vi "Main.vi"() -> ()   [LabVIEW 2018]
uses:
  TypeDefs/Enum_MainQueueElements.ctl
  TypeDefs/Refs_Common.ctl
  TypeDefs/Graph_DataArrayElement.ctl
  <vilib>/event_ctls.llb/eventvkey.ctl
  TypeDefs/TD_Case_SimpleFGVModes.ctl
  TypeDefs/Enum_CmdPromptActions.ctl
  TypeDefs/TD_Case_RecControll_DisableControlls.ctl
  OXYGEN/TypeDefs/Cluster_RawCommData.ctl
  TypeDefs/TD_Case_MeasurementValues.ctl
  OXYGEN/TypeDefs/Enum_ELOGtimeFormats.ctl
  TypeDefs/TD_Case_ELOG-ManageGUI.ctl
  OXYGEN/VIs/Common Commands/SubVIs/GetID.vi
  OXYGEN/VIs/Common Commands/SubVIs/GetSoftwareVersion.vi
  OXYGEN/VIs/Error Handling/SubVIs/ErrorHandling_GetError.vi
  OXYGEN/VIs/Application Control/SubVIs/ApplicationSetup_Load.vi
  OXYGEN/VIs/Recording Control/SubVIs/RecordingControl_SetFileName.vi
  OXYGEN/VIs/Channel List Access/SubVIs/ChannelList_GetNames.vi
  OXYGEN/VIs/Recording Control/SubVIs/RecordingControl_Start.vi
  OXYGEN/VIs/Recording Control/SubVIs/RecordingControl_Pause.vi
  OXYGEN/VIs/Recording Control/SubVIs/RecordingControl_Stop.vi
  OXYGEN/VIs/Measurement Values/SubVIs/AggregationRate_Set.vi
  OXYGEN/VIs/Measurement Values/SubVIs/MeasurementItems_SetChannels.vi
  OXYGEN/VIs/External Data Logging/SubVIs/ELOG_Channels_Set.vi
  OXYGEN/VIs/External Data Logging/SubVIs/ELOG_AggregationPeriod_Set.vi
  OXYGEN/VIs/External Data Logging/SubVIs/ELOG_Calculations_Set.vi
  OXYGEN/VIs/External Data Logging/SubVIs/ELOG_TimestampFormat_Set.vi
  OXYGEN/VIs/External Data Logging/SubVIs/ELOG_Control_Start.vi
  OXYGEN/VIs/External Data Logging/SubVIs/ELOG_Control_Stop.vi
  OXYGEN/VIs/External Data Logging/SubVIs/ELOG_Control_Reset.vi
  OXYGEN.lvlib
panel:
  out "Bool_StatusLED":bool=TRUE
  in  "STR_HostAddress":string
  in  "Button_Disconnect":bool
  in  "Button_Connect":bool
  in  "LBox_ChList":i32(listbox)
  in  "Tab_Selections":T1(tab)
  in  "Indicator_RecordingStatus":u32(colorbox)
  in  "STR_SetupSetFileName":path
  in  "STR_SetupLoadFileName":path
  in  "Button_Identification":bool
  in  "Button_Version":bool
  in  "Button_Reset":bool
  in  "Button_Error":bool
  in  "Button_LoadSetup":bool
  in  "Button_SetFileName":bool
  in  "Button_QuerryChList":bool
  in  "Button_StartRec":bool
  in  "Button_PauseRec":bool
  in  "Button_StopRec":bool
  in  "Button_UsrCmdSet":bool
  in  "STR_UserCommand":string
  in  "Button_AggregationRate":bool
  in  "STR_IN_AggregationRate":dbl=0.001 min=0.001 max=5.0 format="%.3p"
  in  "STR_ChName1":string
  out "Num_ChValue1":dbl format="%04.3g"
  in  "STR_ChName2":string
  out "Num_ChValue2":dbl format="%1.3g"
  in  "STR_ChName3":string
  out "Num_ChValue3":dbl format="%1.3g"
  in  "STR_ChName4":string
  out "Num_ChValue4":dbl format="%.3g"
  in  "STR_ChName5":string
  out "Num_ChValue5":dbl format="%.3g"
  in  "STR_ChName6":string
  out "Num_ChValue6":dbl format="%.3g"
  out "Recorder":T2(graph)
  in  "Button_StartTransfer":bool
  in  "Button_StopTransfer":bool
  in  "STR_LoggingChName3":string
  in  "STR_LoggingChName2":string
  in  "STR_LoggingChName4":string
  in  "STR_LoggingChName5":string
  in  "STR_LoggingChName6":string
  in  "Enum_SelectCalc":u16(ring) items=["AVG", "MIN", "MAX", "RMS"]
  in  "Enum_SelectTimestampFormat":u16(ring) items=["OFF", "REL", "ABS", "ELOG"]
  in  "Num_SetDurationTime":dbl=0.001 min=0.0001 max=30.0 format="%1.3p"
  in  "STR_LoggingChName1":string
  out "Listbox_ChValue":i32(listbox)
  out "RecoderLogging":T2(graph)
  in  "Button_StartBuffer":bool
  in  "Button_FetchData":bool
  in  "Button_StopBuffer":bool
  out "STR_CmdPrompt":string
  # "IP Address/Hostname and Port Number \n                Example:  xxx.xxx.xxx.xxx:Port"
  # "Common Commands"
  # "Setup Managment"
  # "Recording Control"
  # "User Command"
  # "s"
  # "Channel 1"
  # "Channel 3"
  # "Channel 2"
  # "Channel 5"
  # "Channel 4"
  # "Channel 6"
  # "Channel 1"
  # "Channel 2"
  # "Channel 3"
  # "Channel 4"
  # "Channel 5"
  # "Channel 6"
  # "Timestamp"
  # "Calculations"
  # "Period"
  # "s"
  # "Channel 1"
  # "Channel 2"
  # "Channel 3"
  # "Channel 4"
  # "Channel 5"
  # "Channel 6"
  # "Channel 1"
  # "Channel 2"
  # "Channel 3"
  # "Channel 4"
  # "Channel 5"
  # "Channel 6"
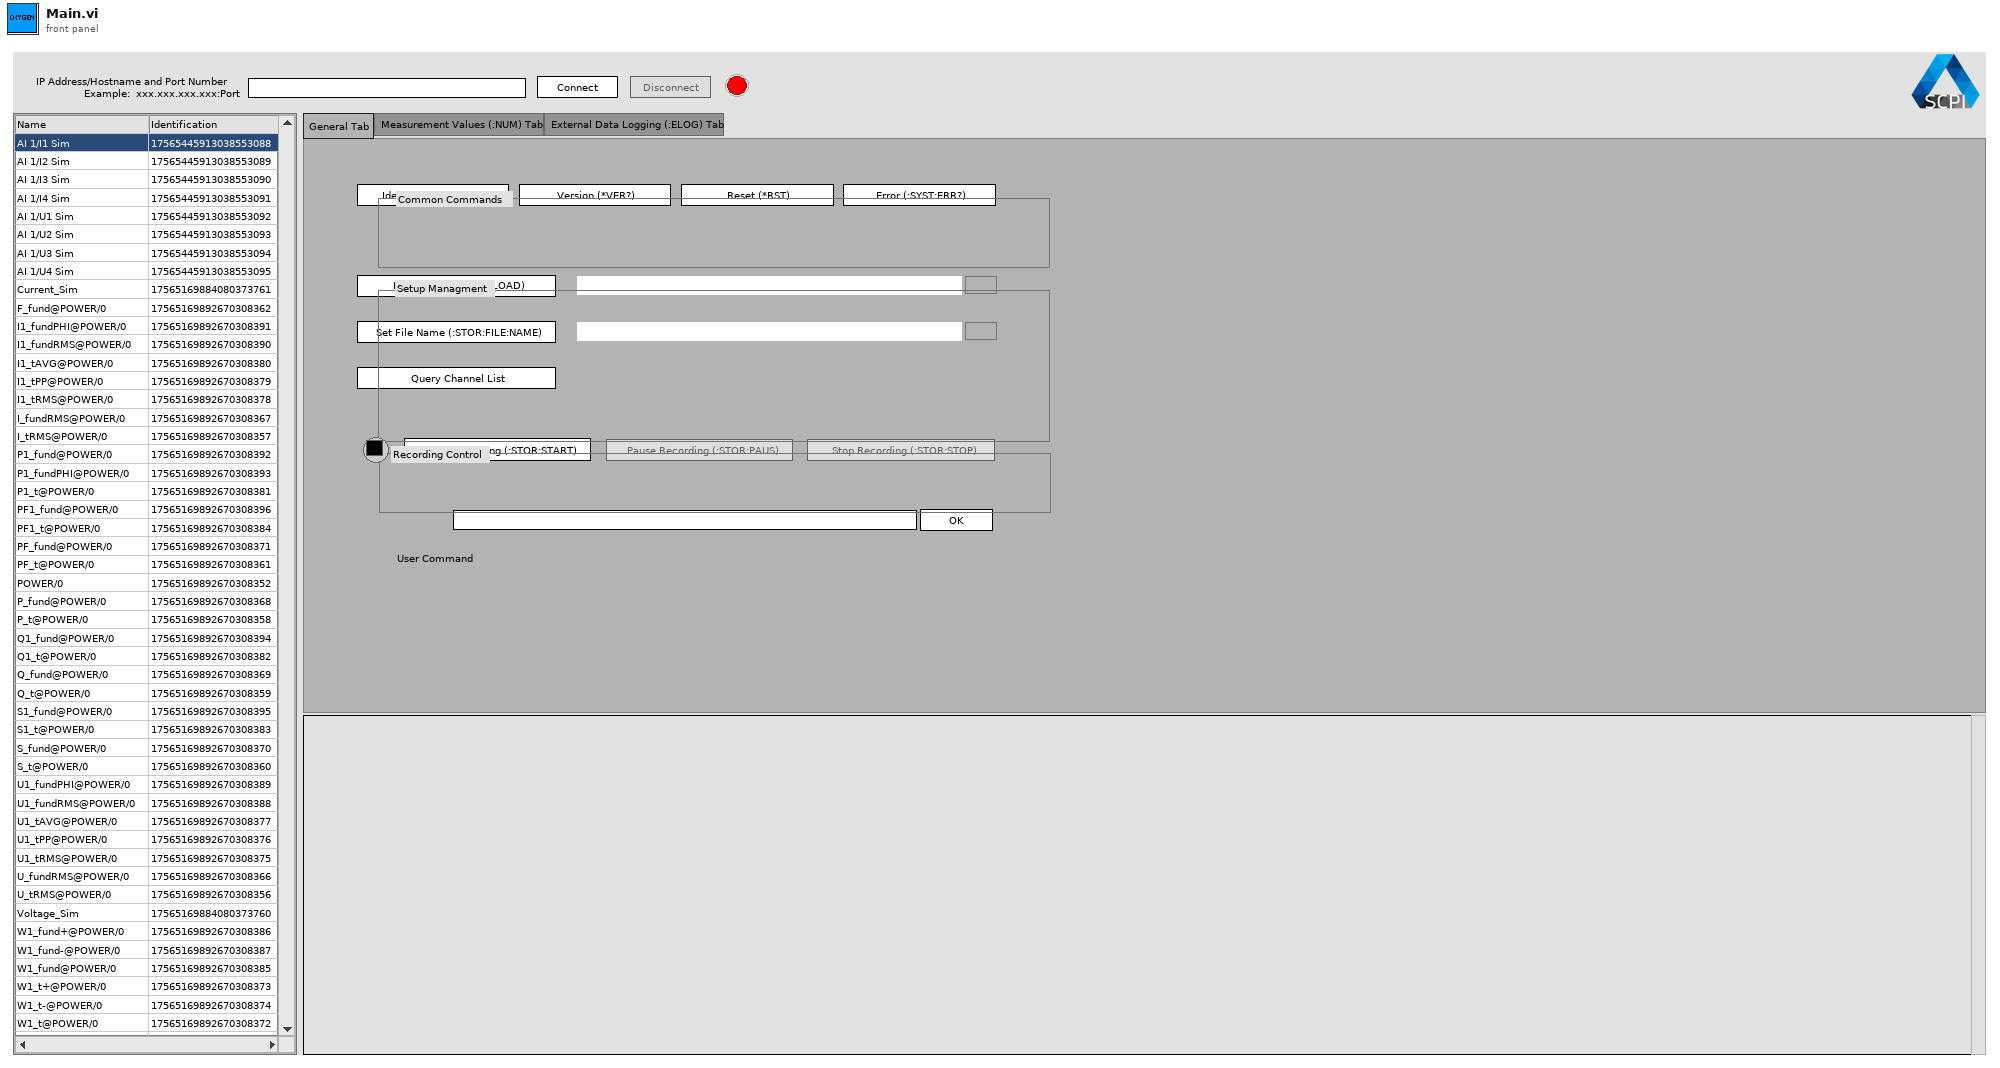
[diagram p1: front panel]
types:
  T1 = enum32{"General Tab", "Measurement Values (:NUM) Tab", "External Data Logging (:ELOG) Tab"}
  T2 = cluster{"Timestamp":timestamp[], "Value":dbl[]}[]
  T3 = typedef "Graph_DataArrayElement.ctl" = cluster{"Timestamp":timestamp[], "Value":dbl[]}
  T4 = typedef "Refs_Common.ctl" = cluster{"LBox_ChList":refnum<vi>, "STR_LoggingChName1":refnum<vi>, "Listbox_ChValue":refnum<vi>, "STR_LoggingChName2":refnum<vi>, "STR_LoggingChName3":refnum<vi>, "STR_LoggingChName4":refnum<vi>, "STR_LoggingChName5":refnum<vi>, "STR_LoggingChName6":refnum<vi>, "OXY_SCPI Ref":refnum<visa-resource-name>, "STR_ChName1":refnum<vi>, "STR_ChName2":refnum<vi>, "STR_ChName3":refnum<vi>, "STR_ChName4":refnum<vi>, "STR_ChName5":refnum<vi>, "STR_ChName6":refnum<vi>, "Enum_SelectTimestampFormat":refnum<vi>, "GRAPH-XY_ELOG":refnum<vi>, "GRAPH-XY_Measurement":refnum<vi>, "Button_StartBuffer":refnum<vi>, "Button_StopBuffer":refnum<vi>, "Button_FetchData":refnum<vi>, "STR_LoggingChName1":refnum<vi>, "STR_LoggingChName2":refnum<vi>, "STR_LoggingChName3":refnum<vi>, "STR_LoggingChName4":refnum<vi>, "STR_LoggingChName5":refnum<vi>, "STR_LoggingChName6":refnum<vi>, "Enum_SelectCalc":refnum<vi>, "Num_SetDurationTime":refnum<vi>, "Button_StopTransfer":refnum<vi>, "Button_StartTransfer":refnum<vi>, "STR_IN_AggregationRate":refnum<vi>, "Button_Disconnect":refnum<vi>, "Button_Connect":refnum<vi>, "Button_StartRec":refnum<vi>, "Button_PauseRec":refnum<vi>, "Button_StopRec":refnum<vi>, "Bool_StatusLED":refnum<vi>, "Indicator_RecordingStatus":refnum<vi>}
  T5 = typedef "Enum_MainQueueElements.ctl" = enum16{"Timeout", "Init", "Button_Identification_Pressed", "Button_Version_Pressed", "Button_Reset_Pressed", "Button_Error_Pressed", "Button_LoadSetup_Pressed", "Button_SetFileName_Pressed", "Button_QuerryChList_Pressed", "Button_StartRec_Pressed", "Button_PauseRec_Pressed", "Button_StopRec_Pressed", "Button_UsrCmdSet_Pressed", "Button_AggregationRate_Pressed", "Button_StartTransfer_Pressed", "Button_StopTransfer_Pressed", "Button_StartBuffer_Pressed", "Button_FetchData_Pressed", "Button_StopBuffer_Pressed", "Button_Connect_Pressed", "Button_Disconnect_Pressed", "NewDragAndDrop", "CloseApp"}
  T6 = typedef "Enum_CmdPromptActions.ctl" = enum16{"Init", "Add", "EditSettings", "Close"}
  T7 = typedef "TD_Case_RecControll_DisableControlls.ctl" = enum16{"Start", "Pause", "Stop"}
  T8 = typedef "OXYGEN.lvlib/Cluster_RawCommData.ctl" = cluster{"send_data":string, "received_data":string}
  T9 = typedef "TD_Case_MeasurementValues.ctl" = enum16{"Init", "Start", "Stop", "ChangeChannel", "Refresh"}
  T10 = typedef "OXYGEN.lvlib/Enum_ELOGtimeFormats.ctl" = enum16{"OFF", "REL", "ELOG", "ABS"}
  T11 = typedef "TD_Case_ELOG-ManageGUI.ctl" = enum16{"Reset", "AddDataToGUI"}
  T12 = enum8{"Enabled", "Disabled", "Disabled and Grayed Out"}
  T13 = typedef "TD_Case_SimpleFGVModes.ctl" = enum16{"Set", "Get"}
  T14 = typedef "OXYGEN.lvlib/Cluster_ChannelList_Names.ctl" = cluster{"ID":string, "Name":string}
  T15 = typedef "eventvkey.ctl" = enum16{"ASCII", "Enter", "Return", "Shift", "Ctrl", "Alt", "Cmd", "Opt", "Caps", "NumLock", "Clear", "Break", "Up", "Down", "Left", "Right", "Insert", "Delete", "Home", "End", "PageUp", "PageDown", "Escape", "Help", "Pause", "ScrollLock", "F1", "F2", "F3", "F4", "F5", "F6", "F7", "F8", "F9", "F10", "F11", "F12", "F13", "F14", "F15", "F16", "F17", "F18", "F19", "F20", "F21", "F22", "F23", "F24", "Play", "VolumeUp", "VolumeDown", "Mute", "Two Byte Char"}
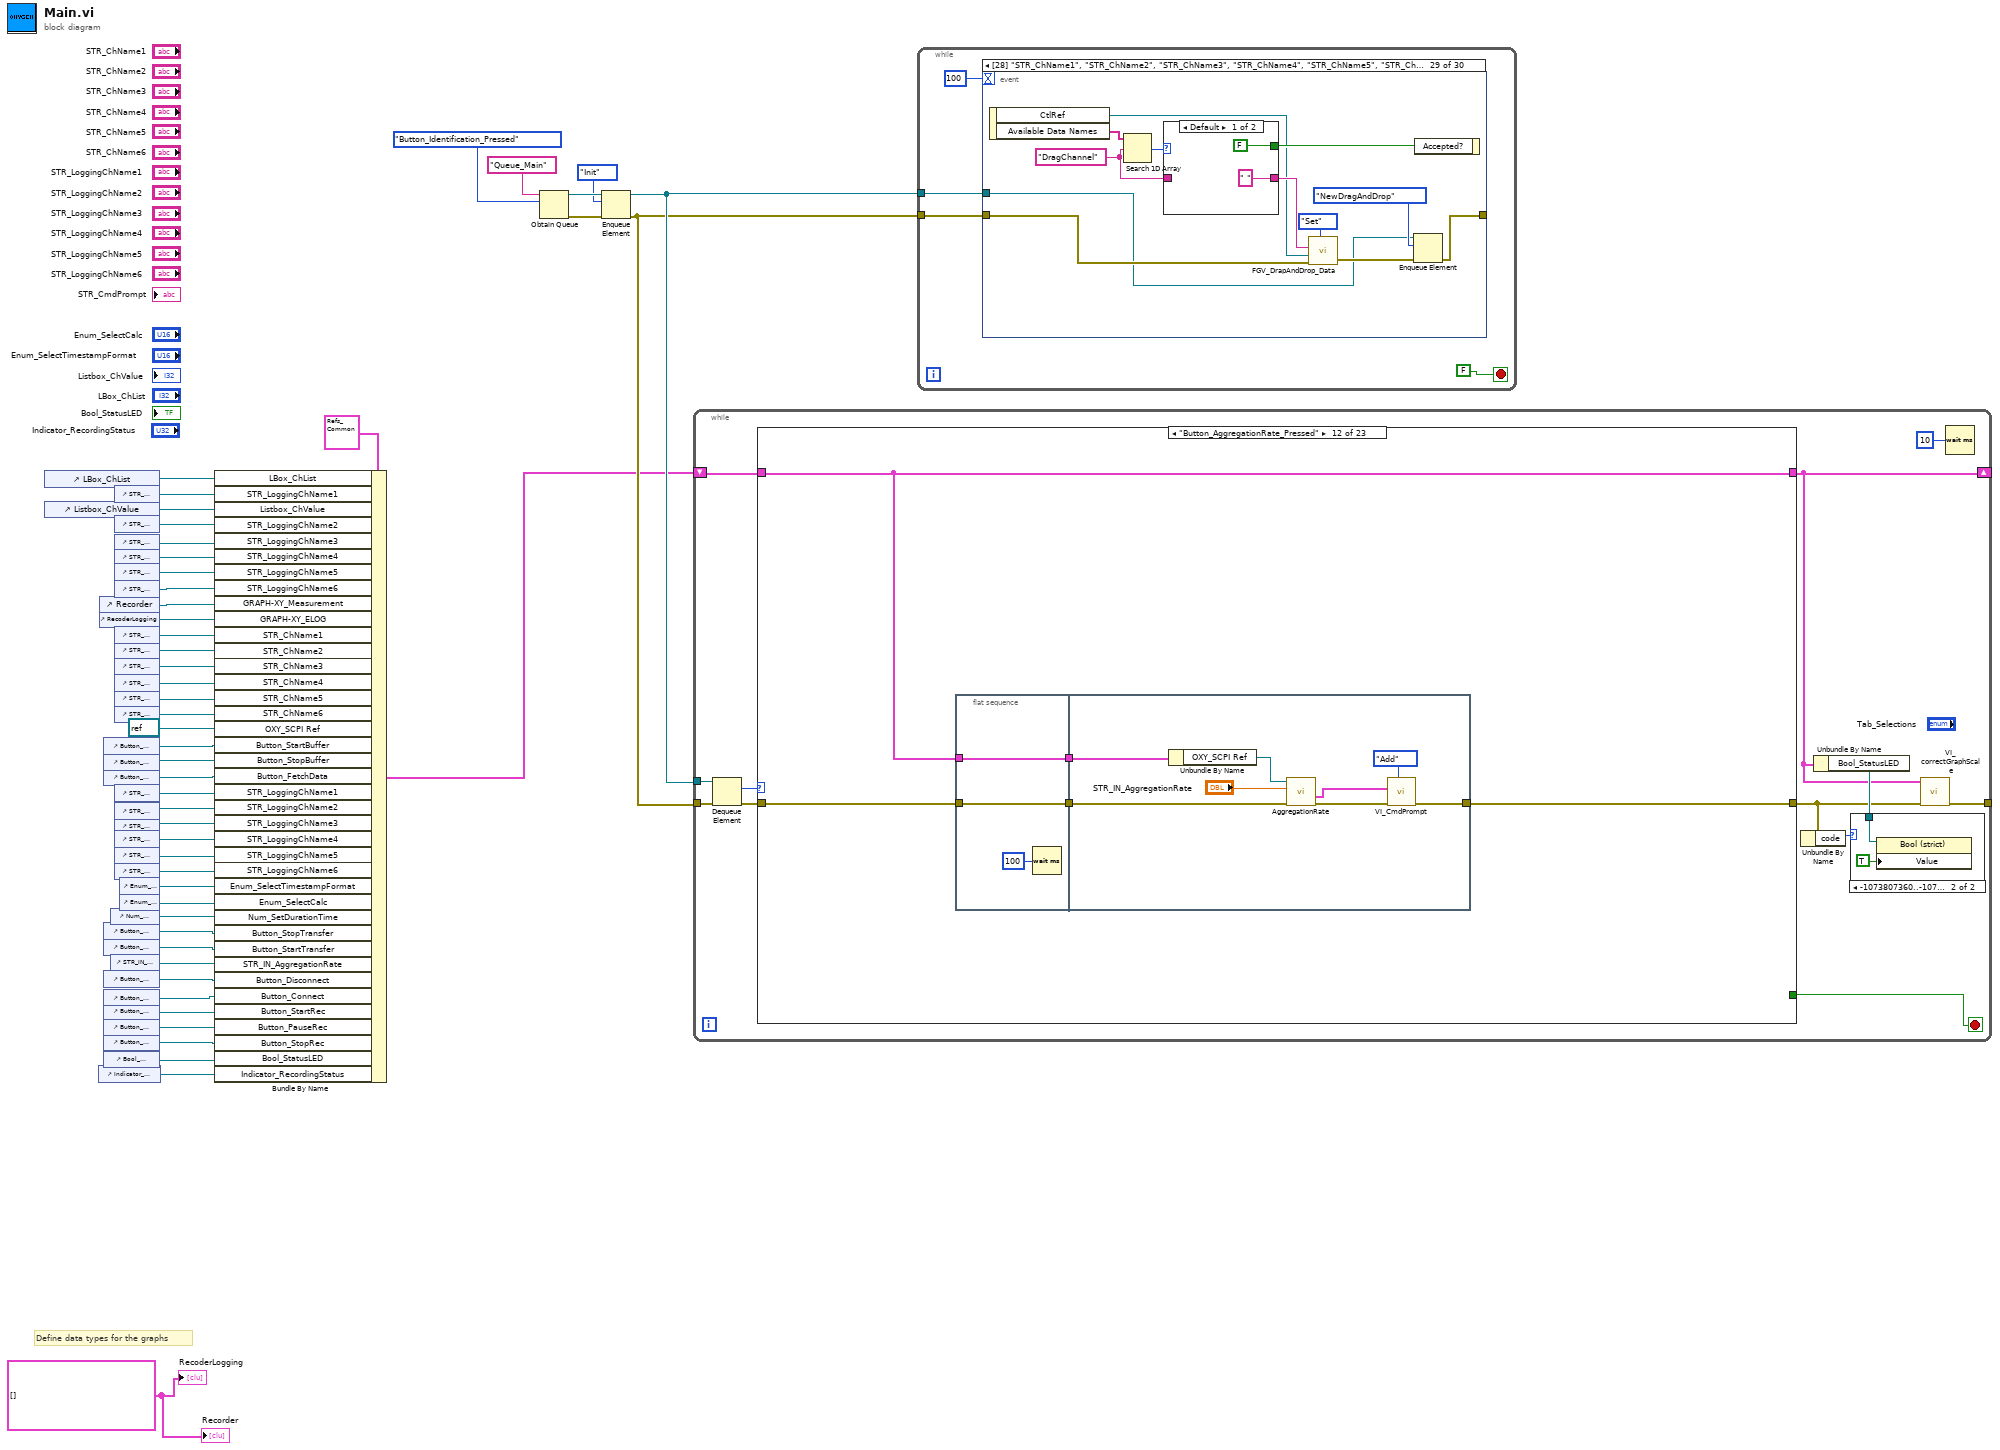
[diagram p0: block diagram]
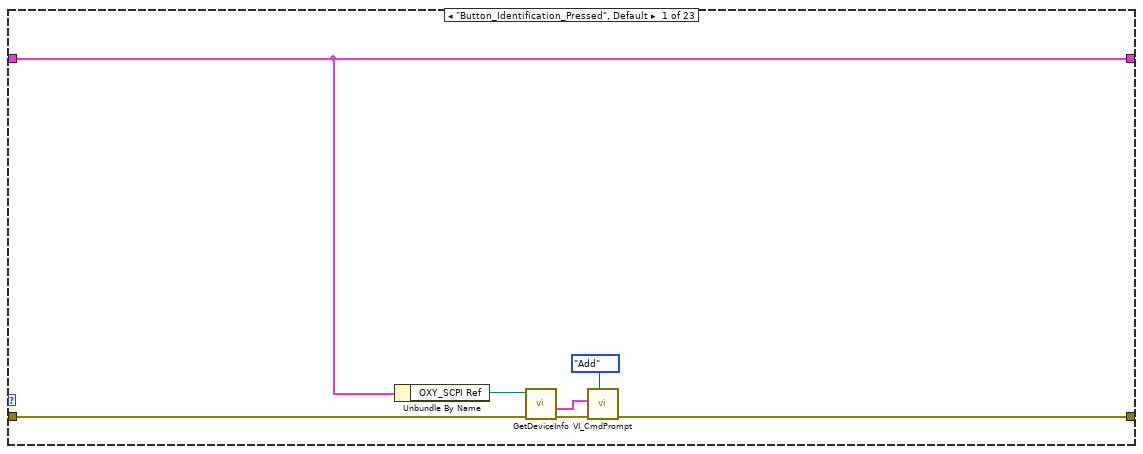
[diagram p3: hidden frame]
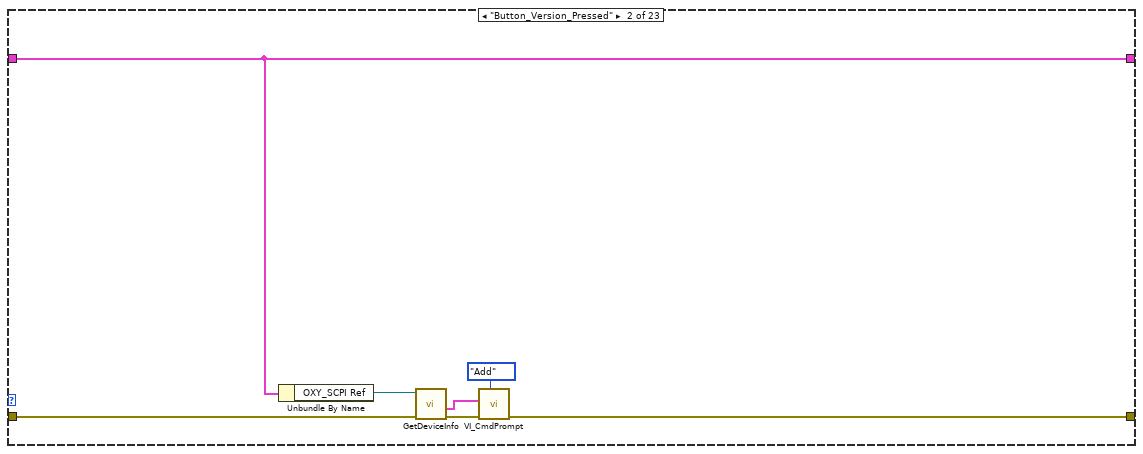
[diagram p4: hidden frame]
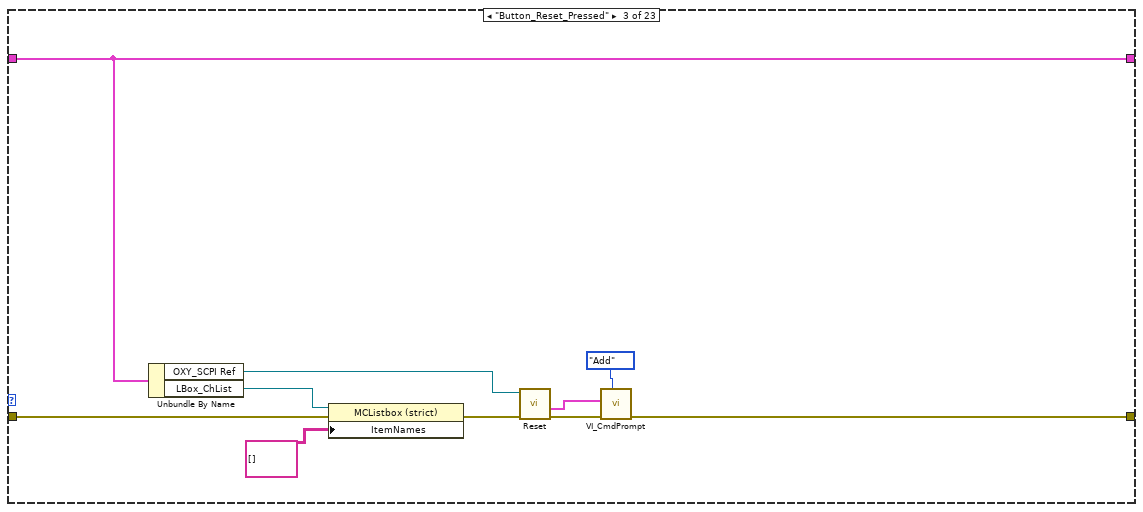
[diagram p5: hidden frame]
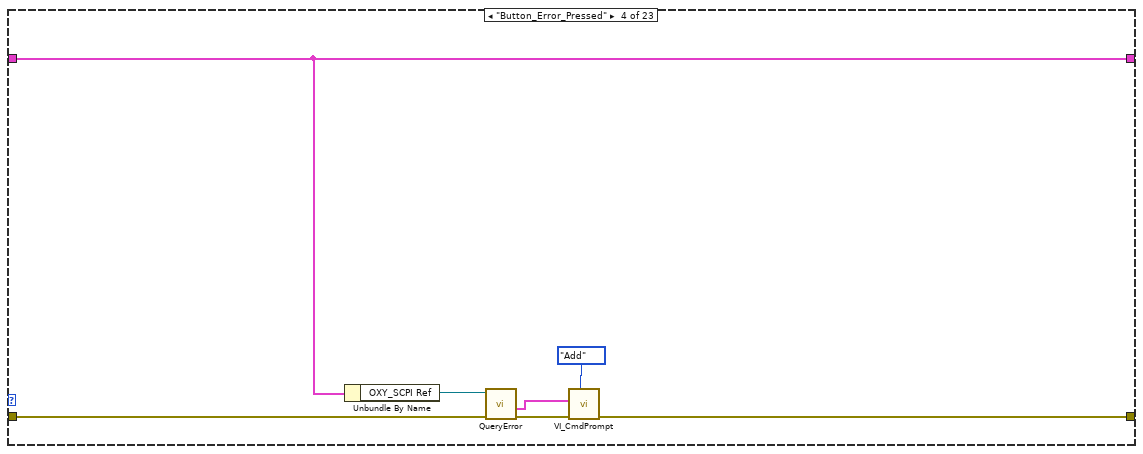
[diagram p6: hidden frame]
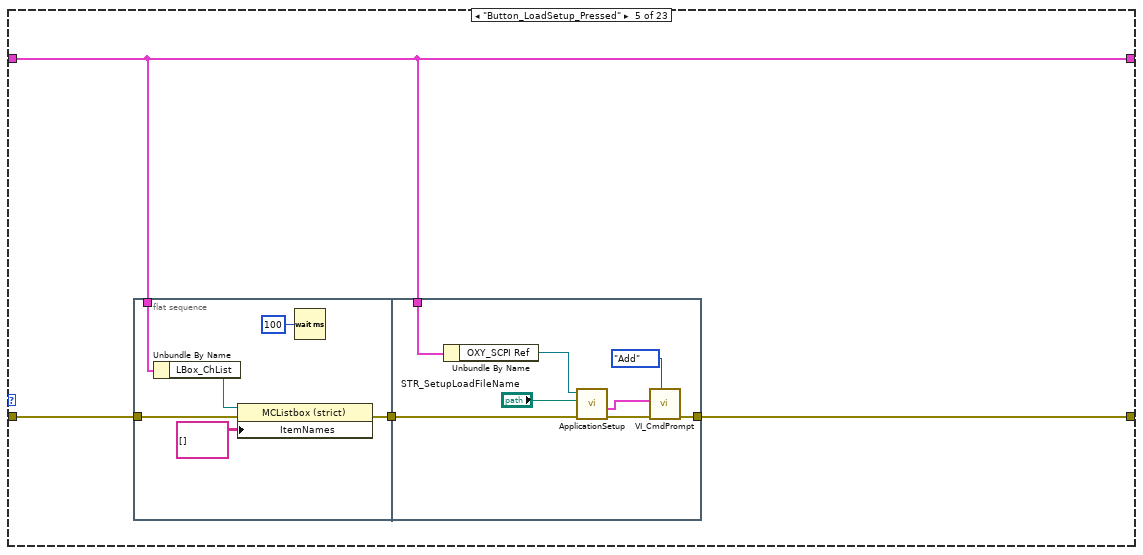
[diagram p7: hidden frame]
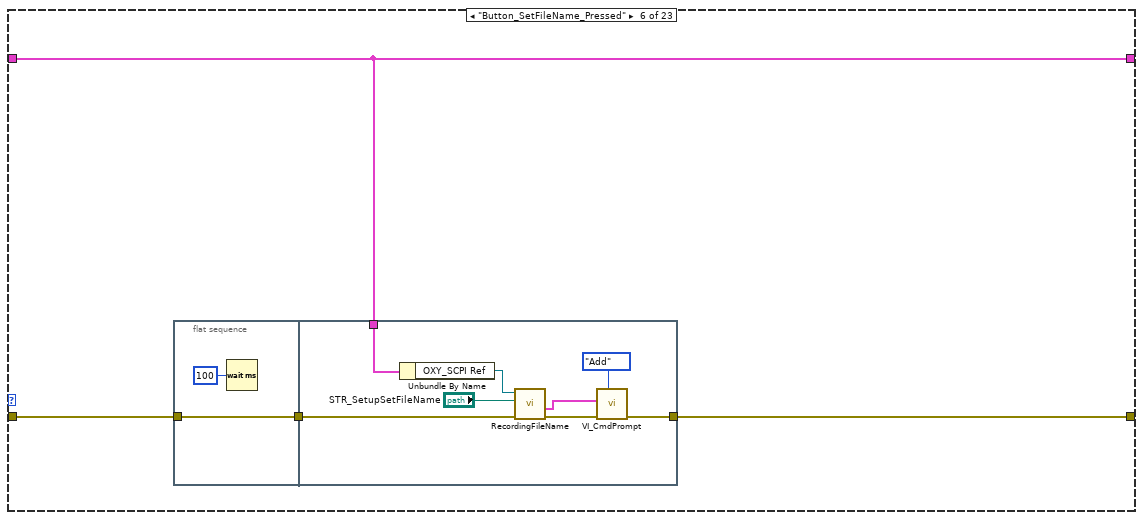
[diagram p8: hidden frame]
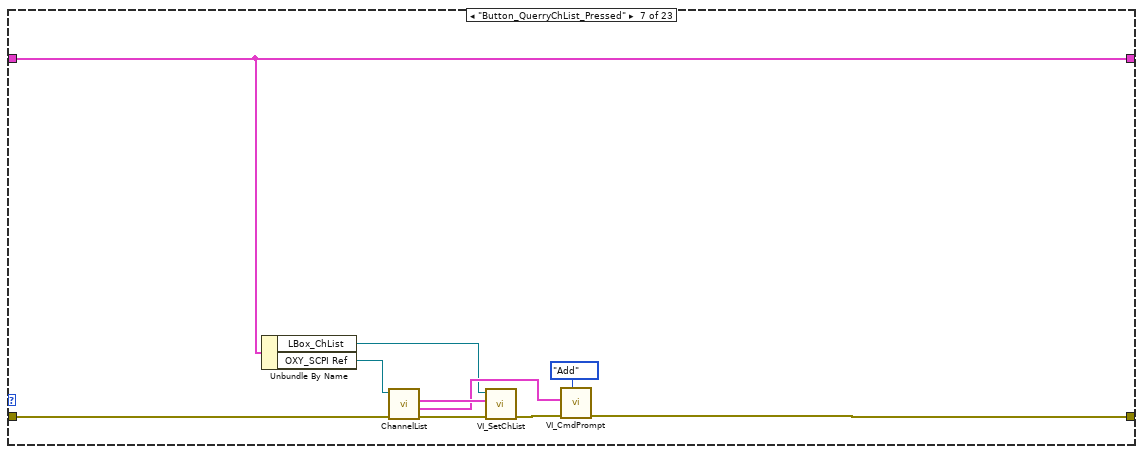
[diagram p9: hidden frame]
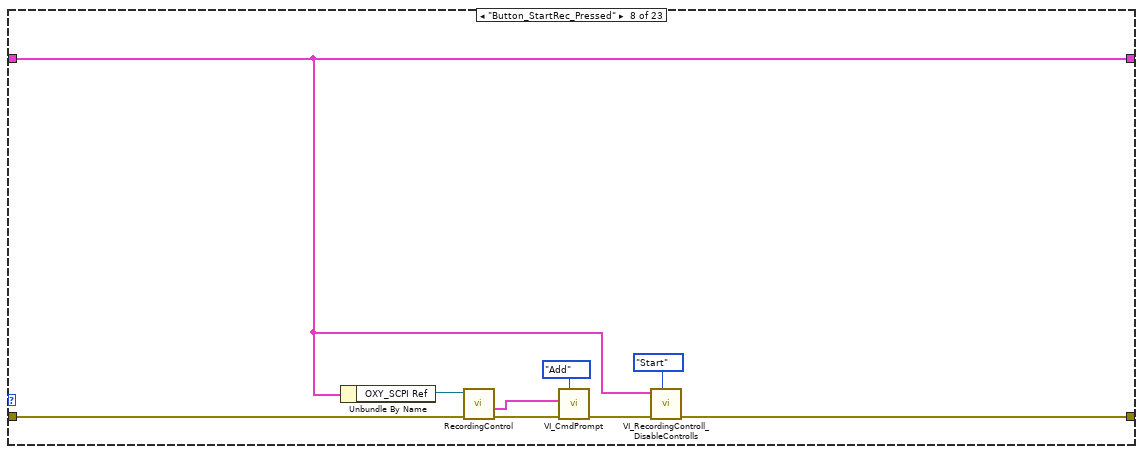
[diagram p10: hidden frame]
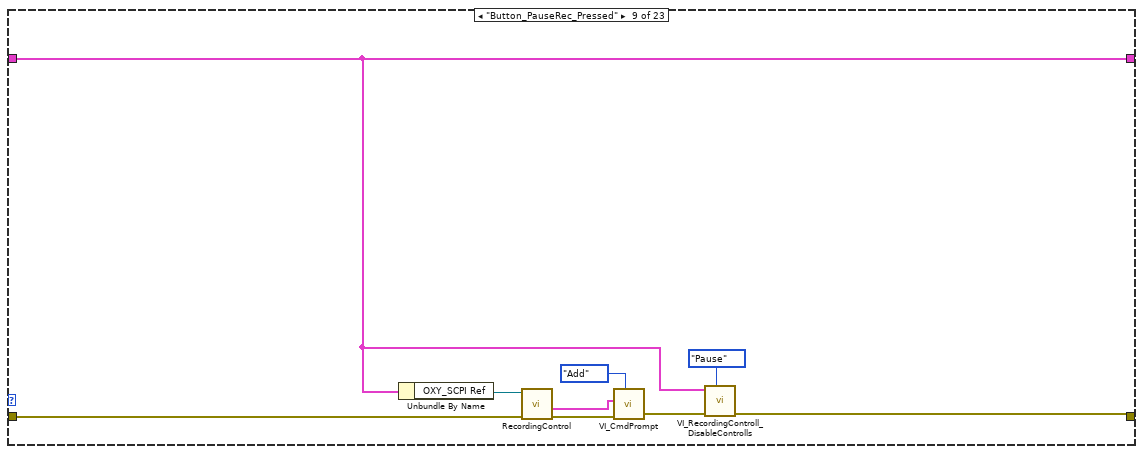
[diagram p11: hidden frame]
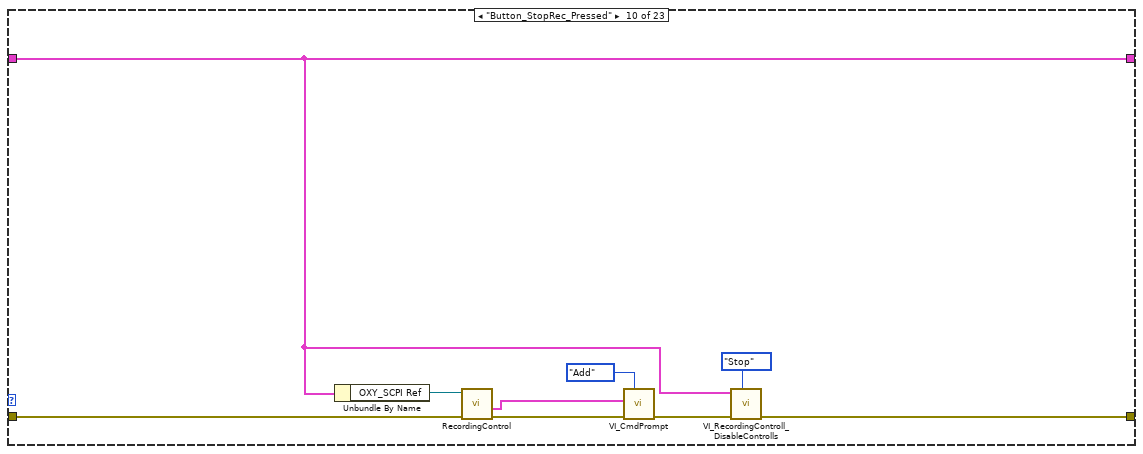
[diagram p12: hidden frame]
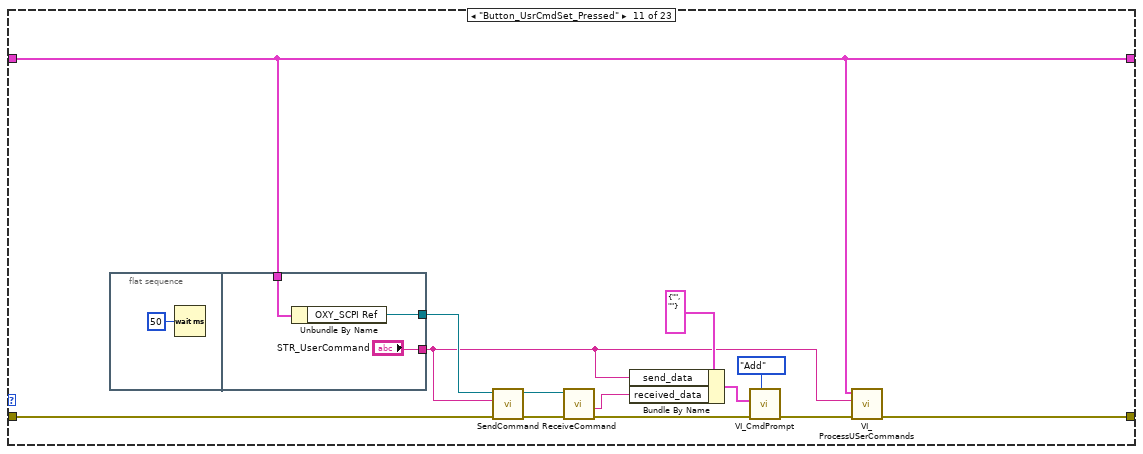
[diagram p13: hidden frame]
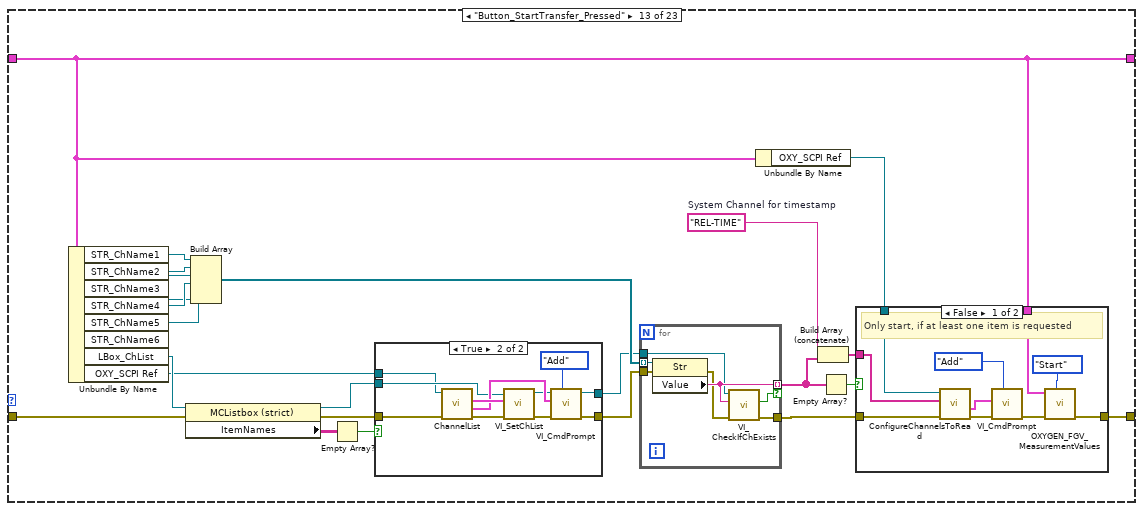
[diagram p14: hidden frame]
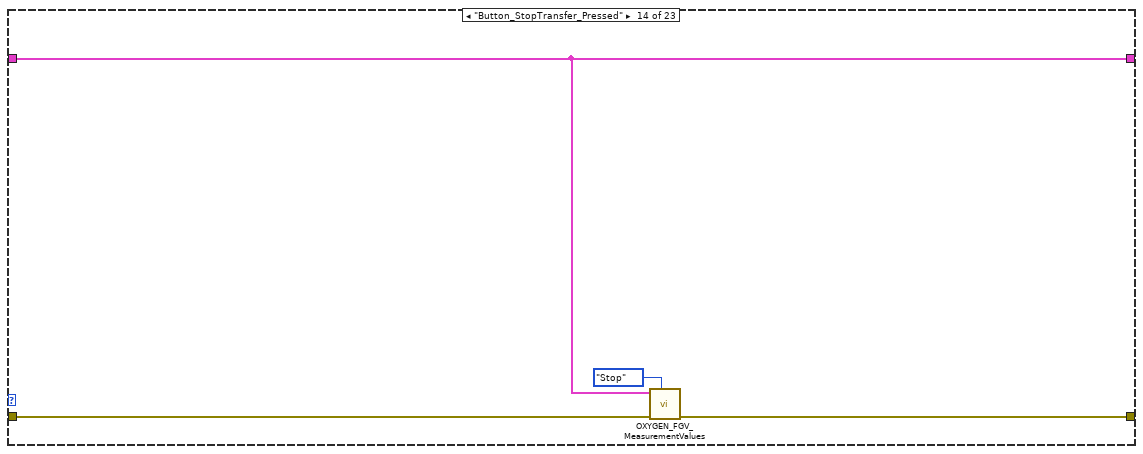
[diagram p17: hidden frame]
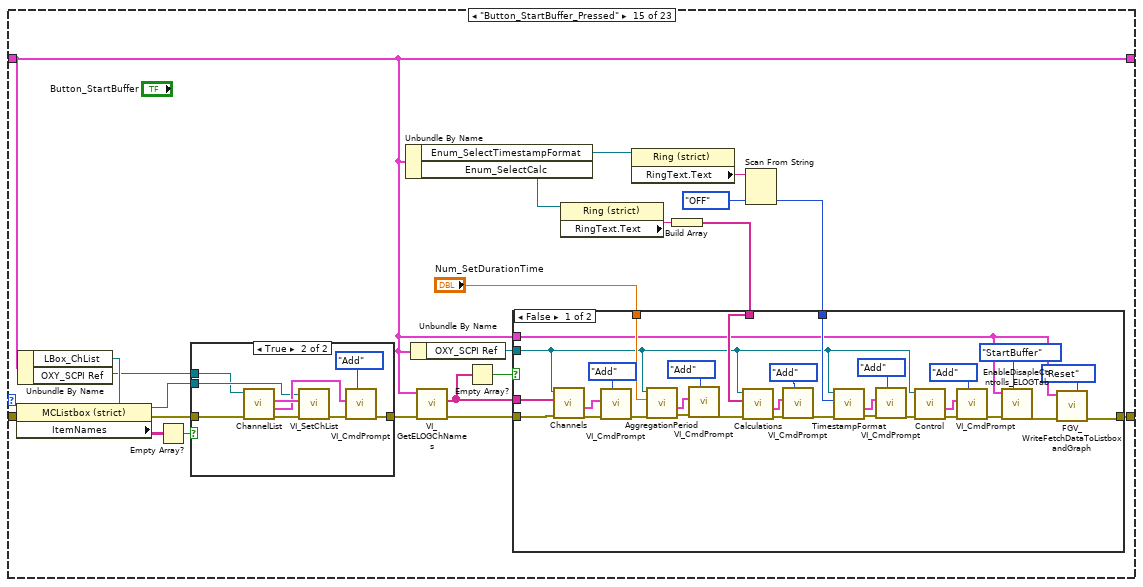
[diagram p18: hidden frame]
diagram:
  w4 = T3[] [] ("Updated Graph Data")
  # "Define data types for the graphs"
  n1 = control-ref of="LBox_ChList"() -> (w29:refnum<vi>)
  n2 = control-ref of="Listbox_ChValue"() -> (w32:refnum<vi>)
  n3 = control-ref of="Indicator_RecordingStatus"() -> (w1:refnum<vi>)
  n4 = control-ref of="Recorder"() -> (w25:refnum<vi>)
  n5 = control-ref of="RecoderLogging"() -> (w3:refnum<vi>)
  n6 = control-ref of="Button_StartBuffer"() -> (w24:refnum<vi>)
  n7 = control-ref of="Button_StopBuffer"() -> (w23:refnum<vi>)
  n8 = control-ref of="Button_FetchData"() -> (w22:refnum<vi>)
  n9 = control-ref of="Button_StopTransfer"() -> (w12:refnum<vi>)
  n10 = control-ref of="Button_StartTransfer"() -> (w11:refnum<vi>)
  n11 = control-ref of="Button_Disconnect"() -> (w9:refnum<vi>)
  n12 = control-ref of="Button_Connect"() -> (w8:refnum<vi>)
  n13 = control-ref of="Button_StartRec"() -> (w7:refnum<vi>)
  n14 = control-ref of="Button_PauseRec"() -> (w6:refnum<vi>)
  n15 = control-ref of="Button_StopRec"() -> (w5:refnum<vi>)
  n16 = control-ref of="Bool_StatusLED"() -> (w2:refnum<vi>)
  n17 = control-ref of="Num_SetDurationTime"() -> (w13:refnum<vi>)
  n18 = control-ref of="STR_IN_AggregationRate"() -> (w10:refnum<vi>)
  n19 = control-ref of="STR_LoggingChName1"() -> (w30:refnum<vi>)
  n20 = control-ref of="STR_LoggingChName2"() -> (w36:refnum<vi>)
  n21 = control-ref of="STR_LoggingChName3"() -> (w35:refnum<vi>)
  n22 = control-ref of="STR_LoggingChName4"() -> (w34:refnum<vi>)
  n23 = control-ref of="STR_LoggingChName5"() -> (w33:refnum<vi>)
  n24 = control-ref of="STR_LoggingChName6"() -> (w31:refnum<vi>)
  n25 = control-ref of="STR_ChName1"() -> (w37:refnum<vi>)
  n26 = control-ref of="STR_ChName2"() -> (w38:refnum<vi>)
  n27 = control-ref of="STR_ChName3"() -> (w39:refnum<vi>)
  n28 = control-ref of="STR_ChName4"() -> (w40:refnum<vi>)
  n29 = control-ref of="STR_ChName5"() -> (w41:refnum<vi>)
  n30 = control-ref of="STR_ChName6"() -> (w42:refnum<vi>)
  n31 = control-ref of="STR_LoggingChName1"() -> (w21:refnum<vi>)
  n32 = control-ref of="STR_LoggingChName2"() -> (w20:refnum<vi>)
  n33 = control-ref of="STR_LoggingChName3"() -> (w19:refnum<vi>)
  n34 = control-ref of="STR_LoggingChName4"() -> (w18:refnum<vi>)
  n35 = control-ref of="STR_LoggingChName5"() -> (w17:refnum<vi>)
  n36 = control-ref of="STR_LoggingChName6"() -> (w16:refnum<vi>)
  n37 = control-ref of="Enum_SelectTimestampFormat"() -> (w15:refnum<vi>)
  n38 = control-ref of="Enum_SelectCalc"() -> (w14:refnum<vi>)
  n39 = Bundle By Name(cluster=T4 {"LBox_ChList"=refnum, "STR_LoggingChName1"=refnum, "Listbox_ChValue"=refnum, "STR_LoggingChName2"=refnum, "STR_LoggingChName3"=refnum, "STR_LoggingChName4"=refnum, "STR_LoggingChName5"=refnum, "STR_LoggingChName6"=refnum, "OXY_SCPI Ref"="TCPIP0::192.168.1.75::10001::SOCKET", "STR_ChName1"=refnum, "STR_ChName2"=refnum, "STR_ChName3"=refnum, "STR_ChName4"=refnum, "STR_ChName5"=refnum, "STR_ChName6"=refnum, "Enum_SelectTimestampFormat"=refnum, "GRAPH-XY_ELOG"=refnum, "GRAPH-XY_Measurement"=refnum, "Button_StartBuffer"=refnum, "Button_StopBuffer"=refnum, "Button_FetchData"=refnum, "STR_LoggingChName1"=refnum, "STR_LoggingChName2"=refnum, "STR_LoggingChName3"=refnum, "STR_LoggingChName4"=refnum, "STR_LoggingChName5"=refnum, "STR_LoggingChName6"=refnum, "Enum_SelectCalc"=refnum, "Num_SetDurationTime"=refnum, "Button_StopTransfer"=refnum, "Button_StartTransfer"=refnum, "STR_IN_AggregationRate"=refnum, "Button_Disconnect"=refnum, "Button_Connect"=refnum, "Button_StartRec"=refnum, "Button_PauseRec"=refnum, "Button_StopRec"=refnum, "Bool_StatusLED"=refnum, "Indicator_RecordingStatus"=refnum} ("Common Refs"), "LBox_ChList"=w29, "STR_LoggingChName1"=w30, "Listbox_ChValue"=w32, "STR_LoggingChName2"=w36, "STR_LoggingChName3"=w35, "STR_LoggingChName4"=w34, "STR_LoggingChName5"=w33, "STR_LoggingChName6"=w31, "GRAPH-XY_Measurement"=w25, "GRAPH-XY_ELOG"=w3, "STR_ChName1"=w37, "STR_ChName2"=w38, "STR_ChName3"=w39, "STR_ChName4"=w40, "STR_ChName5"=w41, "STR_ChName6"=w42, "OXY_SCPI Ref"=refnum<visa-resource-name> refnum, "Button_StartBuffer"=w24, "Button_StopBuffer"=w23, "Button_FetchData"=w22, "STR_LoggingChName1"=w21, "STR_LoggingChName2"=w20, "STR_LoggingChName3"=w19, "STR_LoggingChName4"=w18, "STR_LoggingChName5"=w17, "STR_LoggingChName6"=w16, "Enum_SelectTimestampFormat"=w15, "Enum_SelectCalc"=w14, "Num_SetDurationTime"=w13, "Button_StopTransfer"=w12, "Button_StartTransfer"=w11, "STR_IN_AggregationRate"=w10, "Button_Disconnect"=w9, "Button_Connect"=w8, "Button_StartRec"=w7, "Button_PauseRec"=w6, "Button_StopRec"=w5, "Bool_StatusLED"=w2, "Indicator_RecordingStatus"=w1) -> (w26:T4)
  n40 = Obtain Queue(name (unnamed)="Queue_Main", element data type=Enum_MainQueueElements."Button_Identification_Pressed") -> (queue out=w47:refnum<queue>, error out=w44:errorcluster)  [unwired: 3 in, 1 out]
  n41 = Enqueue Element(queue=w47, element=Enum_MainQueueElements."Init", error in (no error)=w44) -> (queue out=w46:refnum<queue>, error out=w45:errorcluster)  [unwired: 1 in, 1 out]
  n42 = while {
    tunnel: w46 -> [w56]
    shift-right: [w52] -> _
    shift-left: w26 -> [w55]
    tunnel: w45 -> [w60]
    tunnel: [w51] -> _
    stop <- w57 stop-if-true
    n43 = Dequeue Element(queue=w56, error in (no error)=w60) -> (element=w59:T5, error out=w58:errorcluster)  [unwired: 1 in, 2 out]
    n44 = case shown="\"Button_AggregationRate_Pressed\"" w59 {
      tunnel: w58 -> [w67 w74 w78 w91 w97 w114 w133 w144 w150 w161 w176 w183 w203 w254 w256 w328 w337 w350 w385 w390 w411 w424 w430]
      tunnel: [w69 w76 w86 w93 w98 w115 w128 w139 w147 w156 w166 w185 w220 w253 w268 w330 w334 w342 w383 w386 w410 w428 w429] -> w50
      tunnel: w55 -> [w68 w75 w85 w88 w95 w116 w135 w140 w146 w155 w165 w184 w209 w251 w259 w320 w335 w346 w374 w388 w409 w427 w438]
      tunnel: [_ _ _ _ _ _ _ _ _ _ _ _ _ _ _ _ _ _ _ _ _ TRUE _] -> w57
      tunnel: [w68 w75 w85 w88 w95 w116 w135 w140 w146 w155 w165 w184 w209 w251 w259 w320 w335 w343 w378 w388 w409 w427 w438] -> w52
      frame "Button_Identification_Pressed", Default {
        n45 = Unbundle By Name(w68) -> ("OXY_SCPI Ref"=w65:refnum<visa-resource-name>)
        n46 = call-poly "GetDeviceInfo.vi"("Fehler (Eingang, kein Fehler)"=w67, "OXYGEN Ref In"=w65) -> ("Fehler (Ausgang)"=w64:errorcluster, "Raw communication data"=w66:T8)  [unwired: 6 in, 2 out]
        n47 = call "VI_CmdPrompt.vi"("Mode"=Enum_CmdPromptActions."Add", "error in (no error)"=w64, "communication_data"=w66) -> ("error out"=w69:errorcluster)  [unwired: 8 in]
      }
      frame "Button_Version_Pressed" {
        n48 = Unbundle By Name(w75) -> ("OXY_SCPI Ref"=w73:refnum<visa-resource-name>)
        n49 = call-poly "GetDeviceInfo.vi"("Fehler (Eingang, kein Fehler)"=w74, "OXYGEN Ref In"=w73) -> ("Fehler (Ausgang)"=w71:errorcluster, "Raw communication data"=w72:T8)  [unwired: 6 in, 2 out]
        n50 = call "VI_CmdPrompt.vi"("Mode"=Enum_CmdPromptActions."Add", "error in (no error)"=w71, "communication_data"=w72) -> ("error out"=w76:errorcluster)  [unwired: 8 in]
      }
      frame "Button_Reset_Pressed" {
        n51 = Unbundle By Name(w85) -> ("OXY_SCPI Ref"=w80:refnum<visa-resource-name>, "LBox_ChList"=w81:refnum<vi>)
        n52 = property class="MCListbox (strict)"(reference=w81, error in=w78, "ItemNames"=string[][] [] ("Item Names")) -> (error out=w79:errorcluster)  [unwired: 1 out]
        n53 = call "Reset.vi"("Fehler (Eingang, kein Fehler)"=w79, "Referenz_In"=w80) -> ("Fehler (Ausgang)"=w84:errorcluster, "communication_data"=w83:T8)  [unwired: 7 in, 1 out]
        n54 = call "VI_CmdPrompt.vi"("Mode"=Enum_CmdPromptActions."Add", "error in (no error)"=w84, "communication_data"=w83) -> ("error out"=w86:errorcluster)  [unwired: 8 in]
      }
      frame "Button_Error_Pressed" {
        n55 = Unbundle By Name(w88) -> ("OXY_SCPI Ref"=w90:refnum<visa-resource-name>)
        n56 = call-poly "QueryError.vi"("Fehler (Eingang, kein Fehler)"=w91, "Referenz_In"=w90) -> ("Fehler (Ausgang)"=w92:errorcluster, "communication_data"=w89:T8)  [unwired: 6 in, 2 out]
        n57 = call "VI_CmdPrompt.vi"("Mode"=Enum_CmdPromptActions."Add", "error in (no error)"=w92, "communication_data"=w89) -> ("error out"=w93:errorcluster)  [unwired: 8 in]
      }
      frame "Button_LoadSetup_Pressed" {
        n58 = flat-sequence {
          tunnel: w97 -> [w102]
          tunnel: [w101] -> w96
          tunnel: w95 -> [w99]
          tunnel: w95 -> [w111]
          tunnel: [w110] -> w98
          tunnel: w96 -> [w109]
          frame #0 {
            n59 = Unbundle By Name(w99) -> ("LBox_ChList"=w100:refnum<vi>)
            n60 = property class="MCListbox (strict)"(reference=w100, error in=w102, "ItemNames"=string[][] [] ("Item Names")) -> (error out=w101:errorcluster)  [unwired: 1 out]
            n61 = Wait (ms)(milliseconds to wait=u32 100) -> ()  [unwired: 1 out]
          }
          frame #1 {
            n62 = Unbundle By Name(w111) -> ("OXY_SCPI Ref"=w106:refnum<visa-resource-name>)
            n63 = call-poly "ApplicationSetup.vi"("error in (no error)"=w109, "Path"="STR_SetupLoadFileName", "OXYGEN Ref In"=w106) -> ("error out"=w108:errorcluster, "communication_data"=w107:T8)  [unwired: 6 in, 1 out]
            n64 = call "VI_CmdPrompt.vi"("Mode"=Enum_CmdPromptActions."Add", "error in (no error)"=w108, "communication_data"=w107) -> ("error out"=w110:errorcluster)  [unwired: 8 in]
          }
        }
      }
      frame "Button_SetFileName_Pressed" {
        n65 = flat-sequence {
          tunnel: w114 -> [w118]
          tunnel: [w118] -> w113
          tunnel: w116 -> [w125]
          tunnel: [w124] -> w115
          tunnel: w113 -> [w123]
          frame #0 {
            n66 = Wait (ms)(milliseconds to wait=u32 100) -> ()  [unwired: 1 out]
          }
          frame #1 {
            n67 = Unbundle By Name(w125) -> ("OXY_SCPI Ref"=w119:refnum<visa-resource-name>)
            n68 = call-poly "RecordingFileName.vi"("error in (no error)"=w123, "File Name or Path"="STR_SetupSetFileName", "OXY_SCPI Reseource In"=w119) -> ("error out"=w122:errorcluster, "communication_data"=w121:T8)  [unwired: 6 in, 1 out]
            n69 = call "VI_CmdPrompt.vi"("Mode"=Enum_CmdPromptActions."Add", "error in (no error)"=w122, "communication_data"=w121) -> ("error out"=w124:errorcluster)  [unwired: 8 in]
          }
        }
      }
      frame "Button_QuerryChList_Pressed" {
        n70 = Unbundle By Name(w135) -> ("LBox_ChList"=w127:refnum<vi>, "OXY_SCPI Ref"=w134:refnum<visa-resource-name>)
        n71 = call-poly "ChannelList.vi"("error in (no error)"=w133, "OXY_SCPI Reseource In"=w134) -> ("error out"=w132:errorcluster, "communication_data"=w130:T8, "Channel List"=w131:T14[])  [unwired: 6 in, 1 out]
        n72 = call "VI_SetChList.vi"("error in (no error)"=w132, "Channel List"=w131, "ChList_Ref In"=w127) -> ("error out"=w129:errorcluster)  [unwired: 7 in, 1 out]
        n73 = call "VI_CmdPrompt.vi"("Mode"=Enum_CmdPromptActions."Add", "error in (no error)"=w129, "communication_data"=w130) -> ("error out"=w128:errorcluster)  [unwired: 8 in]
      }
      frame "Button_StartRec_Pressed" {
        n74 = Unbundle By Name(w140) -> ("OXY_SCPI Ref"=w142:refnum<visa-resource-name>)
        n75 = call-poly "RecordingControl.vi"("error in (no error)"=w144, "OXY_SCPI Reseource In"=w142) -> ("error out"=w143:errorcluster, "communication_data"=w141:T8)  [unwired: 7 in, 1 out]
        n76 = call "VI_CmdPrompt.vi"("Mode"=Enum_CmdPromptActions."Add", "error in (no error)"=w143, "communication_data"=w141) -> ("error out"=w138:errorcluster)  [unwired: 8 in]
        n77 = call "VI_RecordingControll_DisableControlls.vi"("Mode"=TD_Case_RecControll_DisableControlls."Start", "error in (no error)"=w138, "Common Refs"=w140) -> ("error out"=w139:errorcluster)  [unwired: 8 in]
      }
      frame "Button_PauseRec_Pressed" {
        n78 = Unbundle By Name(w146) -> ("OXY_SCPI Ref"=w151:refnum<visa-resource-name>)
        n79 = call-poly "RecordingControl.vi"("error in (no error)"=w150, "OXY_SCPI Reseource In"=w151) -> ("error out"=w153:errorcluster, "communication_data"=w152:T8)  [unwired: 7 in, 1 out]
        n80 = call "VI_CmdPrompt.vi"("Mode"=Enum_CmdPromptActions."Add", "error in (no error)"=w153, "communication_data"=w152) -> ("error out"=w148:errorcluster)  [unwired: 8 in]
        n81 = call "VI_RecordingControll_DisableControlls.vi"("Mode"=TD_Case_RecControll_DisableControlls."Pause", "error in (no error)"=w148, "Common Refs"=w146) -> ("error out"=w147:errorcluster)  [unwired: 8 in]
      }
      frame "Button_StopRec_Pressed" {
        n82 = Unbundle By Name(w155) -> ("OXY_SCPI Ref"=w160:refnum<visa-resource-name>)
        n83 = call-poly "RecordingControl.vi"("error in (no error)"=w161, "OXY_SCPI Reseource In"=w160) -> ("error out"=w162:errorcluster, "communication_data"=w159:T8)  [unwired: 7 in, 1 out]
        n84 = call "VI_CmdPrompt.vi"("Mode"=Enum_CmdPromptActions."Add", "error in (no error)"=w162, "communication_data"=w159) -> ("error out"=w157:errorcluster)  [unwired: 8 in]
        n85 = call "VI_RecordingControll_DisableControlls.vi"("Mode"=TD_Case_RecControll_DisableControlls."Stop", "error in (no error)"=w157, "Common Refs"=w155) -> ("error out"=w156:errorcluster)  [unwired: 8 in]
      }
      frame "Button_UsrCmdSet_Pressed" {
        n86 = flat-sequence {
          tunnel: w165 -> [w180]
          tunnel: [w179] -> w174
          tunnel: ["STR_UserCommand"] -> w164
          frame #0 {
            n87 = Wait (ms)(milliseconds to wait=u32 50) -> ()  [unwired: 1 out]
          }
          frame #1 {
            n88 = Unbundle By Name(w180) -> ("OXY_SCPI Ref"=w179:refnum<visa-resource-name>)
          }
        }
        n89 = call "SendCommand.vi"("error in (no error)"=w176, "String to Send"=w164, "OXY_SCPI Reseource In"=w174) -> ("error out"=w171:errorcluster, "OXY_SCPI Reseource Out"=w172:refnum<visa-resource-name>)  [unwired: 7 in]
        n90 = call "ReceiveCommand.vi"("error in (no error)"=w171, "OXY_SCPI Reseource In"=w172) -> ("error out"=w169:errorcluster, "received Data with Header"=w167:string)  [unwired: 6 in, 2 out]
        n91 = Bundle By Name(cluster=T8 {"send_data"="", "received_data"=""} ("communication_data"), "send_data"=w164, "received_data"=w167) -> (w168:T8)
        n92 = call "VI_CmdPrompt.vi"("Mode"=Enum_CmdPromptActions."Add", "error in (no error)"=w169, "communication_data"=w168) -> ("error out"=w175:errorcluster)  [unwired: 8 in]
        n93 = call "VI_ProcessUSerCommands.vi"("error in (no error)"=w175, "send command"=w164, "Common Refs"=w165) -> ("error out"=w166:errorcluster)  [unwired: 8 in]
      }
      frame "Button_AggregationRate_Pressed" {
        n94 = flat-sequence {
          tunnel: w183 -> [w187]
          tunnel: w184 -> [w188]
          tunnel: [w188] -> w182
          tunnel: [w187] -> w181
          tunnel: [w195] -> w185
          tunnel: w182 -> [w194]
          tunnel: w181 -> [w193]
          frame #0 {
            n95 = Wait (ms)(milliseconds to wait=u32 100) -> ()  [unwired: 1 out]
          }
          frame #1 {
            n96 = Unbundle By Name(w194) -> ("OXY_SCPI Ref"=w191:refnum<visa-resource-name>)
            n97 = call-poly "AggregationRate.vi"("error in (no error)"=w193, "Aggregation Rate (s) (<0 for NONE)"="STR_IN_AggregationRate", "OXY_SCPI Reseource In"=w191) -> ("error out"=w192:errorcluster, "communication_data"=w189:T8)  [unwired: 6 in, 1 out]
            n98 = call "VI_CmdPrompt.vi"("Mode"=Enum_CmdPromptActions."Add", "error in (no error)"=w192, "communication_data"=w189) -> ("error out"=w195:errorcluster)  [unwired: 8 in]
          }
        }
      }
      frame "Button_StartTransfer_Pressed" {
        w210 = "REL-TIME"  # System Channel for timestamp
        n99 = Unbundle By Name(w209) -> ("STR_ChName1"=w219:refnum<vi>, "STR_ChName2"=w218:refnum<vi>, "STR_ChName3"=w217:refnum<vi>, "STR_ChName4"=w216:refnum<vi>, "STR_ChName5"=w215:refnum<vi>, "STR_ChName6"=w214:refnum<vi>, "LBox_ChList"=w206:refnum<vi>, "OXY_SCPI Ref"=w198:refnum<visa-resource-name>)
        n100 = property class="MCListbox (strict)"(reference=w206, error in=w203) -> (reference out=w204:refnum<vi>, error out=w201:errorcluster, "ItemNames"=w205:string[][])
        n101 = Build Array(w219, w218, w217, w216, w215, w214) -> (w213:refnum<vi>[])
        n102 = Empty Array?(array=w205) -> (empty?=w202:bool)
        n103 = case shown="True" w202 {
          tunnel: w204 -> [w221 w227]
          tunnel: w201 -> [w222 w226]
          tunnel: [w222 w225] -> w200
          tunnel: w198 -> [_ w224]
          tunnel: [w221 w223] -> w197
          frame False {
          }
          frame True {
            n104 = call-poly "ChannelList.vi"("error in (no error)"=w226, "OXY_SCPI Reseource In"=w224) -> ("error out"=w231:errorcluster, "communication_data"=w229:T8, "Channel List"=w230:T14[])  [unwired: 6 in, 1 out]
            n105 = call "VI_SetChList.vi"("error in (no error)"=w231, "Channel List"=w230, "ChList_Ref In"=w227) -> ("error out"=w228:errorcluster, "ChList_Ref Out"=w223:refnum<vi>)  [unwired: 7 in]
            n106 = call "VI_CmdPrompt.vi"("Mode"=Enum_CmdPromptActions."Add", "error in (no error)"=w228, "communication_data"=w229) -> ("error out"=w225:errorcluster)  [unwired: 8 in]
          }
        }
        n107 = for {
          tunnel: w213 -> [w250] mode=indexing
          tunnel: [w249] -> w207 mode=indexing if=w248
          tunnel: w200 -> [w246]
          tunnel: [w245] -> w199
          tunnel: w197 -> [w244]
          n108 = property class="Str"(reference=w250, error in=w246) -> (error out=w247:errorcluster, "Value"=w249:string)  [unwired: 1 out]
          n109 = call "VI_CheckIfChExists.vi"("error in (no error)"=w247, "Channel Name To Check"=w249, "ChList_Ref In"=w244) -> ("error out"=w245:errorcluster, "Channel Exists"=w248:bool)  [unwired: 6 in, 1 out]
        }
        n110 = Unbundle By Name(w209) -> ("OXY_SCPI Ref"=w212:refnum<visa-resource-name>)
        n111 = Build Array (concatenate)(w210, w207) -> (w211:string[])
        n112 = Empty Array?(array=w207) -> (empty?=w208:bool)
        n113 = case shown="False" w208 {
          tunnel: [w242 w243] -> w220
          tunnel: w212 -> [w236 _]
          tunnel: w199 -> [w235 w243]
          tunnel: w211 -> [w234 _]
          tunnel: w209 -> [w233 _]
          frame False {
            # "Only start, if at least one item is requested"
            n114 = call-poly "ConfigureChannelsToRead.vi"("error in (no error)"=w235, "Channel Name List"=w234, "OXY_SCPI Reseource In"=w236) -> ("error out"=w239:errorcluster, "communication_data"=w240:T8)  [unwired: 6 in, 1 out]
            n115 = call "VI_CmdPrompt.vi"("Mode"=Enum_CmdPromptActions."Add", "error in (no error)"=w239, "communication_data"=w240) -> ("error out"=w238:errorcluster)  [unwired: 8 in]
            n116 = call "OXYGEN_FGV_MeasurementValues.vi"("Mode"=TD_Case_MeasurementValues."Start", "error in (no error)"=w238, "Common Refs"=w233) -> ("error in (no error)"=w242:errorcluster)  [unwired: 7 in, 1 out]
          }
          frame True {
          }
        }
      }
      frame "Button_StopTransfer_Pressed" {
        n117 = call "OXYGEN_FGV_MeasurementValues.vi"("Mode"=TD_Case_MeasurementValues."Stop", "error in (no error)"=w254, "Common Refs"=w251) -> ("error in (no error)"=w253:errorcluster)  [unwired: 7 in, 1 out]
      }
      frame "Button_StartBuffer_Pressed" {
        n118 = Unbundle By Name(w259) -> ("LBox_ChList"=w258:refnum<vi>, "OXY_SCPI Ref"=w257:refnum<visa-resource-name>)
        n119 = property class="MCListbox (strict)"(reference=w258, error in=w256) -> (reference out=w262:refnum<vi>, error out=w255:errorcluster, "ItemNames"=w263:string[][])
        n120 = Empty Array?(array=w263) -> (empty?=w261:bool)
        n121 = case shown="True" w261 {
          tunnel: w262 -> [_ w281]
          tunnel: w255 -> [w277 w280]
          tunnel: [w277 w279] -> w260
          tunnel: w257 -> [_ w278]
          frame False {
          }
          frame True {
            n122 = call-poly "ChannelList.vi"("error in (no error)"=w280, "OXY_SCPI Reseource In"=w278) -> ("error out"=w285:errorcluster, "communication_data"=w283:T8, "Channel List"=w284:T14[])  [unwired: 6 in, 1 out]
            n123 = call "VI_SetChList.vi"("error in (no error)"=w285, "Channel List"=w284, "ChList_Ref In"=w281) -> ("error out"=w282:errorcluster)  [unwired: 7 in, 1 out]
            n124 = call "VI_CmdPrompt.vi"("Mode"=Enum_CmdPromptActions."Add", "error in (no error)"=w282, "communication_data"=w283) -> ("error out"=w279:errorcluster)  [unwired: 8 in]
          }
        }
        n125 = Unbundle By Name(w259) -> ("Enum_SelectTimestampFormat"=w265:refnum<vi>, "Enum_SelectCalc"=w264:refnum<vi>)
        n126 = Unbundle By Name(w259) -> ("OXY_SCPI Ref"=w269:refnum<visa-resource-name>)
        n127 = call "VI_GetELOGChNames.vi"("error in (no error)"=w260, "Common Refs"=w259) -> ("error out"=w276:errorcluster, "ChNames (Array)"=w266:string[])  [unwired: 7 in, 1 out]
        n128 = Empty Array?(array=w266) -> (empty?=w267:bool)
        n129 = property class="Ring (strict)"(reference=w264) -> ("RingText.Text"=w273:string)  [unwired: 1 in, 2 out]
        n130 = property class="Ring (strict)"(reference=w265) -> ("RingText.Text"=w271:string)  [unwired: 1 in, 2 out]
        n131 = Build Array(w273) -> (w274:string[])
        n132 = Scan From String "Scan From String"(input string=w271, default 1=Enum_ELOGtimeFormats."OFF" ("Timestamp Format")) -> (output 1=w270:T10)  [unwired: 3 in, 3 out]
        n133 = case shown="False" w267 {
          tunnel: w266 -> [w311 _]
          tunnel: w276 -> [w302 w318]
          tunnel: "Num_SetDurationTime" -> [w309 _]
          tunnel: w274 -> [w307 _]
          tunnel: w270 -> [w304 _]
          tunnel: w269 -> [w287 _]
          tunnel: [w290 w318] -> w268
          tunnel: w259 -> [w288 _]
          frame False {
            n134 = call-poly "Channels.vi"("error in (no error)"=w302, "Channel Name List"=w311, "OXY_SCPI Reseource In"=w287) -> ("error out"=w292:errorcluster, "communication_data"=w310:T8)  [unwired: 6 in, 1 out]
            n135 = call "VI_CmdPrompt.vi"("Mode"=Enum_CmdPromptActions."Add", "error in (no error)"=w292, "communication_data"=w310) -> ("error out"=w301:errorcluster)  [unwired: 8 in]
            n136 = call-poly "AggregationPeriod.vi"("error in (no error)"=w301, "Period Duration (s)"=w309, "OXY_SCPI Reseource In"=w287) -> ("error out"=w293:errorcluster, "communication_data"=w308:T8)  [unwired: 6 in, 1 out]
            n137 = call "VI_CmdPrompt.vi"("Mode"=Enum_CmdPromptActions."Add", "error in (no error)"=w293, "communication_data"=w308) -> ("error out"=w294:errorcluster)  [unwired: 8 in]
            n138 = call-poly "Calculations.vi"("error in (no error)"=w294, "Calculation Mode"=w307, "OXY_SCPI Reseource In"=w287) -> ("error out"=w295:errorcluster, "communication_data"=w306:T8)  [unwired: 6 in, 1 out]
            n139 = call "VI_CmdPrompt.vi"("Mode"=Enum_CmdPromptActions."Add", "error in (no error)"=w295, "communication_data"=w306) -> ("error out"=w296:errorcluster)  [unwired: 8 in]
            n140 = call-poly "TimestampFormat.vi"("error in (no error)"=w296, "Timestamp Format"=w304, "OXY_SCPI Reseource In"=w287) -> ("error out"=w297:errorcluster, "communication_data"=w305:T8)  [unwired: 6 in, 1 out]
            n141 = call "VI_CmdPrompt.vi"("Mode"=Enum_CmdPromptActions."Add", "error in (no error)"=w297, "communication_data"=w305) -> ("error out"=w298:errorcluster)  [unwired: 8 in]
            n142 = call-poly "Control.vi"("error in (no error)"=w298, "OXY_SCPI Reseource In"=w287) -> ("error out"=w299:errorcluster, "communication_data"=w303:T8)  [unwired: 7 in, 1 out]
            n143 = call "VI_CmdPrompt.vi"("Mode"=Enum_CmdPromptActions."Add", "error in (no error)"=w299, "communication_data"=w303) -> ("error out"=w300:errorcluster)  [unwired: 8 in]
            n144 = call "EnableDisapleControlls_ELOGTab.vi"("Enum"=enum16{"StartBuffer", "StopBuffer"}."StartBuffer", "error in (no error)"=w300, "Common Refs"=w288) -> ("error out"=w289:errorcluster)  [unwired: 8 in]
            n145 = call "FGV_WriteFetchDataToListboxandGraph.vi"("Mode"=TD_Case_ELOG-ManageGUI."Reset", "error in (no error)"=w289, "Common Refs"=w288) -> ("error out"=w290:errorcluster)  [unwired: 8 in]
          }
          frame True {
          }
        }
      }
      frame "Button_FetchData_Pressed" {
        w323 = u32 500  # Num_Records (0 for all)
        n146 = Unbundle By Name(w320) -> ("OXY_SCPI Ref"=w326:refnum<visa-resource-name>)
        n147 = call "FetchData.vi"("error in (no error)"=w328, "Num_Records (0 for all)"=w323, "OXY_SCPI Reseource In"=w326) -> ("error out"=w327:errorcluster, "communication_data"=w325:T8, "Raw Data Stream"=w324:string)  [unwired: 5 in, 1 out]
        n148 = Unbundle By Name(w320) -> ("Listbox_ChValue"=w319:refnum<vi>)
        n149 = call "VI_CmdPrompt.vi"("Mode"=Enum_CmdPromptActions."Add", "error in (no error)"=w327, "communication_data"=w325) -> ("error out"=w329:errorcluster)  [unwired: 8 in]
        n150 = call "FGV_WriteFetchDataToListboxandGraph.vi"("Mode"=TD_Case_ELOG-ManageGUI."AddDataToGUI", "error in (no error)"=w327, "FetchDataString"=w324, "Common Refs"=w320) -> ("error out"=w321:errorcluster)  [unwired: 7 in]
        n151 = call "VI_ScrollMCListboxDown.vi"("error in (no error)"=w321, "MCListbox ref"=w319) -> ("error out"=w322:errorcluster)  [unwired: 8 in, 1 out]
        n152 = Merge Errors(w329, w322) -> (w330:errorcluster)
      }
      frame "Button_StopBuffer_Pressed" {
        n153 = Unbundle By Name(w335) -> ("OXY_SCPI Ref"=w336:refnum<visa-resource-name>)
        n154 = call-poly "Control.vi"("error in (no error)"=w337, "OXY_SCPI Reseource In"=w336) -> ("error out"=w339:errorcluster, "communication_data"=w338:T8)  [unwired: 7 in, 1 out]
        n155 = call "VI_CmdPrompt.vi"("Mode"=Enum_CmdPromptActions."Add", "error in (no error)"=w339, "communication_data"=w338) -> ("error out"=w333:errorcluster)  [unwired: 8 in]
        n156 = call "EnableDisapleControlls_ELOGTab.vi"("Enum"=enum16{"StartBuffer", "StopBuffer"}."StopBuffer", "error in (no error)"=w333, "Common Refs"=w335) -> ("error out"=w334:errorcluster)  [unwired: 8 in]
      }
      frame "Button_Connect_Pressed" {
        n157 = flat-sequence {
          tunnel: w350 -> [w369]
          tunnel: [w369] -> w349
          tunnel: [w371] -> w345
          tunnel: [w370] -> w344
          tunnel: w349 -> [w372]
          frame #0 {
            n158 = Wait (ms)(milliseconds to wait=u32 100) -> ()  [unwired: 1 out]
          }
          frame #1 {
            n159 = call "Connect.vi"("error in (no error)"=w372, "OXY_SCPI TCP-IP address"="STR_HostAddress") -> ("error out"=w371:errorcluster, "OXY_SCPI Reseource Out"=w370:refnum<visa-resource-name>)  [unwired: 8 in]
          }
        }
        n160 = Unbundle By Name(w346) -> ("Bool_StatusLED"=w348:refnum<vi>)
        n161 = Unbundle By Name(w345) -> ("status"=w347:bool)
        n162 = property class="Bool (strict)"(reference=w348, "Value"=w347) -> ()  [unwired: 1 in, 2 out]
        n163 = case shown="No Error" w345 {
          selector: w345 -> [w353 w367]
          tunnel: [w356 w367] -> w342
          tunnel: w346 -> [w354 w366]
          tunnel: [w361 w366] -> w343
          tunnel: w344 -> [w357 _]
          frame No Error {
            n164 = Unbundle By Name(w354) -> ("Button_Disconnect"=w365:refnum<vi>, "Button_Connect"=w364:refnum<vi>)
            n165 = property class="Bool"(reference=w365, error in=w353, "DisabledEnum"=T12."Enabled" ("Disabled")) -> (error out=w352:errorcluster)  [unwired: 1 out]
            n166 = property class="Bool"(reference=w364, error in=w352, "DisabledEnum"=T12."Disabled and Grayed Out" ("Disabled")) -> (error out=w351:errorcluster)  [unwired: 1 out]
            n167 = call-poly "Control.vi"("error in (no error)"=w351, "OXY_SCPI Reseource In"=w357) -> ("error out"=w359:errorcluster, "communication_data"=w360:T8, "OXY_SCPI Reseource Out"=w355:refnum<visa-resource-name>)  [unwired: 7 in]
            n168 = Bundle By Name(cluster=w354, "OXY_SCPI Ref"=w355) -> (w361:T4)
            n169 = call "VI_CmdPrompt.vi"("Mode"=Enum_CmdPromptActions."Add", "error in (no error)"=w359, "communication_data"=w360) -> ("error out"=w356:errorcluster)  [unwired: 8 in]
          }
          frame Error {
          }
        }
      }
      frame "Button_Disconnect_Pressed" {
        n170 = Unbundle By Name(w374) -> ("Bool_StatusLED"=w376:refnum<vi>)
        n171 = Unbundle By Name(w374) -> ("Button_Disconnect"=w380:refnum<vi>, "Button_Connect"=w379:refnum<vi>, "OXY_SCPI Ref"=w384:refnum<visa-resource-name>)
        n172 = property class="Bool (strict)"(reference=w376, "Value"=TRUE) -> ()  [unwired: 1 in, 2 out]
        n173 = call "Disconnect.vi"("error in (no error)"=w385, "OXY_SCPI Reseource Out"=w384) -> ("error out"=w383:errorcluster)  [unwired: 9 in]
        n174 = property class="Bool"(reference=w379, "DisabledEnum"=T12."Enabled" ("Disabled")) -> ()  [unwired: 1 in, 2 out]
        n175 = property class="Bool"(reference=w380, "DisabledEnum"=T12."Disabled and Grayed Out" ("Disabled")) -> ()  [unwired: 1 in, 2 out]
        n176 = Bundle By Name(cluster=w374, "OXY_SCPI Ref"=refnum<visa-resource-name> refnum) -> (w378:T4)
      }
      frame "Init" {
        n177 = control-ref of="This VI"() -> (w393:refnum<vi>)
        n178 = invoke class="VI" method="Default Vals.Reinit All"(reference=w393, error in=w390) -> (error out=w389:errorcluster)  [unwired: 1 in, 2 out]
        n179 = control-ref of="STR_CmdPrompt"() -> (w404:refnum<vi>)
        n180 = call "EnableDisapleControlls_ELOGTab.vi"("Enum"=enum16{"StartBuffer", "StopBuffer"}."StopBuffer", "error in (no error)"=w389, "Common Refs"=w388) -> ("error out"=w397:errorcluster)  [unwired: 8 in]
        n181 = call "VI_CmdPrompt.vi"("Mode"=Enum_CmdPromptActions."Init", "error in (no error)"=w397, "Activate?"=TRUE, "STR_CmdPrompt_Ref"=w404) -> ("error out"=w402:errorcluster)  [unwired: 7 in]
        n182 = call "OXYGEN_FGV_MeasurementValues.vi"("Mode"=TD_Case_MeasurementValues."Init", "error in (no error)"=w402, "Common Refs"=w388) -> ("error in (no error)"=w401:errorcluster)  [unwired: 7 in, 1 out]
        n183 = call "FGV_WriteFetchDataToListboxandGraph.vi"("Mode"=TD_Case_ELOG-ManageGUI."Reset", "error in (no error)"=w401, "Common Refs"=w388) -> ("error out"=w396:errorcluster)  [unwired: 8 in]
        n184 = call "InitControlls.vi"("error in (no error)"=w396, "Common Refs"=w388) -> ("error out"=w391:errorcluster)  [unwired: 9 in]
        n185 = call "VI_RecordingControll_DisableControlls.vi"("Mode"=TD_Case_RecControll_DisableControlls."Stop", "error in (no error)"=w391, "Common Refs"=w388) -> ("error out"=w387:errorcluster)  [unwired: 8 in]
        n186 = Unbundle By Name(w388) -> ("Bool_StatusLED"=w395:refnum<vi>)
        n187 = property class="Bool (strict)"(reference=w395, error in=w387, "Value"=TRUE) -> (error out=w386:errorcluster)  [unwired: 1 out]
      }
      frame "Timeout" {
        # "In this case refresh gui elements"
        n188 = Unbundle By Name(w409) -> ("OXY_SCPI Ref"=w408:refnum<visa-resource-name>)
        n189 = Not Equal?(x=w408, y=refnum<visa-resource-name> refnum ("OXY_SCPI Ref")) -> (x != y?=w406:bool)
        n190 = case shown="True" w406 {
          tunnel: w411 -> [w412 w423]
          tunnel: [w412 w413] -> w410
          tunnel: w409 -> [_ w414]
          frame False {
          }
          frame True {
            n191 = call "OXYGEN_FGV_MeasurementValues.vi"("Mode"=TD_Case_MeasurementValues."Refresh", "error in (no error)"=w423, "Common Refs"=w414) -> ("error in (no error)"=w413:errorcluster, "Value List"=w422:dbl[])  [unwired: 7 in]
            n192 = Index Array(array=w422) -> (element #1=→"Num_ChValue1":dbl, element #2=→"Num_ChValue2":dbl, element #3=→"Num_ChValue3":dbl, element #4=→"Num_ChValue4":dbl, element #5=→"Num_ChValue5":dbl, element #6=→"Num_ChValue6":dbl)  [unwired: 6 in]
          }
        }
      }
      frame "CloseApp" {
        n193 = Unbundle By Name(w427) -> ("OXY_SCPI Ref"=w425:refnum<visa-resource-name>)
        n194 = call "Disconnect.vi"("error in (no error)"=w424, "OXY_SCPI Reseource Out"=w425) -> ("error out"=w428:errorcluster)  [unwired: 9 in]
      }
      frame "NewDragAndDrop" {
        n195 = call "FGV_DrapAndDrop_Data.vi"("Modes"=TD_Case_SimpleFGVModes."Get", "error in (no error)"=w430) -> ("error out"=w436:errorcluster, "Target String Element Ref Out"=w435:refnum<vi>, "Channel Name Out"=w431:string)  [unwired: 7 in]
        n196 = property class="Str"(reference=w435, error in=w436) -> (reference out=w434:refnum<vi>, error out=w433:errorcluster, "DisabledEnum"=w432:T12)
        n197 = case shown="\"Enabled\"" w432 {
          tunnel: w434 -> [w442 _]
          tunnel: w433 -> [w441 w443]
          tunnel: w431 -> [w440 _]
          tunnel: [w439 w443] -> w429
          frame "Enabled" {
            # "Write drag and drop data\n(ch. name) to controll"
            n198 = property class="Str"(reference=w442, error in=w441, "Value"=w440) -> (error out=w439:errorcluster)  [unwired: 1 out]
          }
          frame "Disabled", Default {
            # "Do not place drag and drop data (ch name) if controll is diabled"
          }
        }
      }
    }
    n199 = Unbundle By Name(w50) -> ("code"=w53:i32)
    n200 = Unbundle By Name(w52) -> ("Bool_StatusLED"=w54:refnum<vi>)
    n201 = case shown="-1073807360..-1073807192" w53 {
      tunnel: w54 -> [_ w63]
      frame Default {
      }
      frame -1073807360..-1073807192 {
        n202 = property class="Bool (strict)"(reference=w63, "Value"=TRUE) -> ()  [unwired: 1 in, 2 out]
      }
    }
    n203 = call "VI_correctGraphScale.vi"("error in (no error)"=w50, "Common Refs in"=w52) -> ("error out"=w51:errorcluster)  [unwired: 9 in]
    n204 = Wait (ms)(milliseconds to wait=u32 10) -> ()  [unwired: 1 out]
  }
  n205 = while {
    tunnel: w46 -> [w447]
    tunnel: w45 -> [w446]
    stop <- FALSE stop-if-true
    n206 = event shown="[28] \"STR_ChName1\", \"STR_ChName2\", \"STR_ChName3\", \"STR_ChName4\", \"STR_ChName5\", \"STR_ChName6\", \"STR_LoggingChName1\", \"STR_LoggingChName2\", \"STR_LoggingChName3\", \"STR_LoggingChName4\", \"STR_LoggingChName5\", \"STR_LoggingChName6\": Drop" {
      selector: _ -> [_ _ _ _ _ _ _ _ _ _ _ _ _ _ _ _ _ _ _ _ _ _ _ _ _ _ _ _ _ _]
      dyn-events: _ -> [_ _ _ _ _ _ _ _ _ _ _ _ _ _ _ _ _ _ _ _ _ _ _ _ _ _ _ _ _ _]
      timeout: 100 -> [_ _ _ _ _ _ _ _ _ _ _ _ _ _ _ _ _ _ _ _ _ _ _ _ _ _ _ _ _ _]
      tunnel: w447 -> [w448 w455 w458 w462 w466 w470 w474 w488 w492 _ w505 w509 w513 w517 w521 w525 w529 w543 w557 w561 w565 w569 w573 w577 w581 w595 _ _ w611 w631]
      tunnel: w446 -> [w451 w453 w457 w461 w465 w469 w472 w487 w491 _ w504 w508 w512 w516 w520 w524 w528 w544 w556 w560 w564 w568 w572 w576 w580 w594 _ _ w613 w629]
      tunnel: [w450 w452 w456 w460 w464 w468 w473 w486 _ _ w503 w507 w511 w515 w519 w523 w527 w541 w555 w559 w563 w567 w571 w575 w579 w593 _ _ w612 _] -> _
      event Timeout {
        n207 = event-data() -> ()  [unwired: 1 in, 3 out]
        n208 = Enqueue Element(queue=w448, element=Enum_MainQueueElements."Timeout", error in (no error)=w451) -> (error out=w450:errorcluster)  [unwired: 1 in, 2 out]
      }
      event "Button_Identification": Value Change {
        n209 = event-data() -> ()  [unwired: 1 in, 2 out]
        n210 = Enqueue Element(queue=w455, element=Enum_MainQueueElements."Button_Identification_Pressed", error in (no error)=w453) -> (error out=w452:errorcluster)  [unwired: 1 in, 2 out]
      }
      event "Button_Version": Value Change {
        n211 = event-data() -> ()  [unwired: 1 in, 3 out]
        n212 = Enqueue Element(queue=w458, element=Enum_MainQueueElements."Button_Version_Pressed", error in (no error)=w457) -> (error out=w456:errorcluster)  [unwired: 1 in, 2 out]
      }
      event "Button_Reset": Value Change {
        n213 = event-data() -> ()  [unwired: 1 in, 3 out]
        n214 = Enqueue Element(queue=w462, element=Enum_MainQueueElements."Button_Reset_Pressed", error in (no error)=w461) -> (error out=w460:errorcluster)  [unwired: 1 in, 2 out]
      }
      event "Button_Error": Value Change {
        n215 = event-data() -> ()  [unwired: 1 in, 2 out]
        n216 = Enqueue Element(queue=w466, element=Enum_MainQueueElements."Button_Error_Pressed", error in (no error)=w465) -> (error out=w464:errorcluster)  [unwired: 1 in, 2 out]
      }
      event "Button_LoadSetup": Value Change {
        n217 = event-data() -> ()  [unwired: 1 in, 4 out]
        n218 = Enqueue Element(queue=w470, element=Enum_MainQueueElements."Button_LoadSetup_Pressed", error in (no error)=w469) -> (error out=w468:errorcluster)  [unwired: 1 in, 2 out]
      }
      event "STR_SetupLoadFileName": Key Down {
        n219 = event-data() -> ("VKey"=w478:T15)  [unwired: 1 in, 1 out]
        n220 = Equal?(x=w478, y=eventvkey."Enter") -> (x = y?=w476:bool)
        n221 = Equal?(x=w478, y=eventvkey."Return") -> (x = y?=w477:bool)
        n222 = Or(x=w477, y=w476) -> (x .or. y?=w475:bool)
        n223 = case shown="True" w475 {
          tunnel: w474 -> [_ w485]
          tunnel: [w481 w484] -> w473
          tunnel: w472 -> [w481 w483]
          frame False {
          }
          frame True {
            n224 = Enqueue Element(queue=w485, element=Enum_MainQueueElements."Button_LoadSetup_Pressed", error in (no error)=w483) -> (error out=w484:errorcluster)  [unwired: 1 in, 2 out]
          }
        }
      }
      event "Button_SetFileName": Value Change {
        n225 = event-data() -> ()  [unwired: 1 in, 4 out]
        n226 = Enqueue Element(queue=w488, element=Enum_MainQueueElements."Button_SetFileName_Pressed", error in (no error)=w487) -> (error out=w486:errorcluster)  [unwired: 1 in, 2 out]
      }
      event "STR_SetupSetFileName": Key Down {
        n227 = event-data() -> ("VKey"=w490:T15)  [unwired: 1 in]
        n228 = Equal?(x=w490, y=eventvkey."Enter") -> (x = y?=w494:bool)
        n229 = Equal?(x=w490, y=eventvkey."Return") -> (x = y?=w495:bool)
        n230 = Or(x=w495, y=w494) -> (x .or. y?=w493:bool)
        n231 = case shown="True" w493 {
          tunnel: w492 -> [_ w501]
          tunnel: [w498 w500] -> _
          tunnel: w491 -> [w498 w499]
          frame False {
          }
          frame True {
            n232 = Enqueue Element(queue=w501, element=Enum_MainQueueElements."Button_SetFileName_Pressed", error in (no error)=w499) -> (error out=w500:errorcluster)  [unwired: 1 in, 2 out]
          }
        }
      }
      event "STR_SetupLoadFileName": Value Change {
        n233 = event-data() -> ()  [unwired: 1 in, 6 out]
      }
      event "Button_QuerryChList": Value Change {
        n234 = event-data() -> ()  [unwired: 1 in, 4 out]
        n235 = Enqueue Element(queue=w505, element=Enum_MainQueueElements."Button_QuerryChList_Pressed", error in (no error)=w504) -> (error out=w503:errorcluster)  [unwired: 1 in, 2 out]
      }
      event "Button_StartRec": Value Change {
        n236 = event-data() -> ()  [unwired: 1 in, 3 out]
        n237 = Enqueue Element(queue=w509, element=Enum_MainQueueElements."Button_StartRec_Pressed", error in (no error)=w508) -> (error out=w507:errorcluster)  [unwired: 1 in, 2 out]
      }
      event "Button_PauseRec": Value Change {
        n238 = event-data() -> ()  [unwired: 1 in, 5 out]
        n239 = Enqueue Element(queue=w513, element=Enum_MainQueueElements."Button_PauseRec_Pressed", error in (no error)=w512) -> (error out=w511:errorcluster)  [unwired: 1 in, 2 out]
      }
      event "Button_StopRec": Value Change {
        n240 = event-data() -> ()  [unwired: 1 in, 4 out]
        n241 = Enqueue Element(queue=w517, element=Enum_MainQueueElements."Button_StopRec_Pressed", error in (no error)=w516) -> (error out=w515:errorcluster)  [unwired: 1 in, 2 out]
      }
      event "Button_UsrCmdSet": Value Change {
        n242 = event-data() -> ()  [unwired: 1 in, 4 out]
        n243 = Enqueue Element(queue=w521, element=Enum_MainQueueElements."Button_UsrCmdSet_Pressed", error in (no error)=w520) -> (error out=w519:errorcluster)  [unwired: 1 in, 2 out]
      }
      event "Button_AggregationRate": Value Change {
        n244 = event-data() -> ()  [unwired: 1 in, 3 out]
        n245 = Enqueue Element(queue=w525, element=Enum_MainQueueElements."Button_AggregationRate_Pressed", error in (no error)=w524) -> (error out=w523:errorcluster)  [unwired: 1 in, 2 out]
      }
      event "STR_UserCommand": Key Down {
        n246 = event-data() -> ("VKey"=w530:T15)  [unwired: 1 in]
        n247 = Equal?(x=w530, y=eventvkey."Enter") -> (x = y?=w532:bool)
        n248 = Equal?(x=w530, y=eventvkey."Return") -> (x = y?=w533:bool)
        n249 = Or(x=w533, y=w532) -> (x .or. y?=w531:bool)
        n250 = case shown="True" w531 {
          tunnel: w529 -> [_ w539]
          tunnel: [w536 w538] -> w527
          tunnel: w528 -> [w536 w537]
          frame False {
          }
          frame True {
            n251 = Enqueue Element(queue=w539, element=Enum_MainQueueElements."Button_UsrCmdSet_Pressed", error in (no error)=w537) -> (error out=w538:errorcluster)  [unwired: 1 in, 2 out]
          }
        }
      }
      event "STR_IN_AggregationRate": Key Down {
        n252 = event-data() -> ("VKey"=w542:T15)  [unwired: 1 in]
        n253 = Equal?(x=w542, y=eventvkey."Enter") -> (x = y?=w546:bool)
        n254 = Equal?(x=w542, y=eventvkey."Return") -> (x = y?=w547:bool)
        n255 = Or(x=w547, y=w546) -> (x .or. y?=w545:bool)
        n256 = case shown="True" w545 {
          tunnel: w543 -> [_ w554]
          tunnel: [w550 w553] -> w541
          tunnel: w544 -> [w550 w552]
          frame False {
          }
          frame True {
            n257 = Enqueue Element(queue=w554, element=Enum_MainQueueElements."Button_AggregationRate_Pressed", error in (no error)=w552) -> (error out=w553:errorcluster)  [unwired: 1 in, 2 out]
          }
        }
      }
      event "Button_StartTransfer": Value Change {
        n258 = event-data() -> ()  [unwired: 1 in, 3 out]
        n259 = Enqueue Element(queue=w557, element=Enum_MainQueueElements."Button_StartTransfer_Pressed", error in (no error)=w556) -> (error out=w555:errorcluster)  [unwired: 1 in, 2 out]
      }
      event "Button_StopTransfer": Value Change {
        n260 = event-data() -> ()  [unwired: 1 in, 3 out]
        n261 = Enqueue Element(queue=w561, element=Enum_MainQueueElements."Button_StopTransfer_Pressed", error in (no error)=w560) -> (error out=w559:errorcluster)  [unwired: 1 in, 2 out]
      }
      event "Button_StartBuffer": Value Change {
        n262 = event-data() -> ()  [unwired: 1 in, 3 out]
        n263 = Enqueue Element(queue=w565, element=Enum_MainQueueElements."Button_StartBuffer_Pressed", error in (no error)=w564) -> (error out=w563:errorcluster)  [unwired: 1 in, 2 out]
      }
      event "Button_FetchData": Value Change {
        n264 = event-data() -> ()  [unwired: 1 in, 3 out]
        n265 = Enqueue Element(queue=w569, element=Enum_MainQueueElements."Button_FetchData_Pressed", error in (no error)=w568) -> (error out=w567:errorcluster)  [unwired: 1 in, 2 out]
      }
      event "Button_StopBuffer": Value Change {
        n266 = event-data() -> ()  [unwired: 1 in, 3 out]
        n267 = Enqueue Element(queue=w573, element=Enum_MainQueueElements."Button_StopBuffer_Pressed", error in (no error)=w572) -> (error out=w571:errorcluster)  [unwired: 1 in, 2 out]
      }
      event "Button_Connect": Value Change {
        n268 = event-data() -> ()  [unwired: 1 in, 3 out]
        n269 = Enqueue Element(queue=w577, element=Enum_MainQueueElements."Button_Connect_Pressed", error in (no error)=w576) -> (error out=w575:errorcluster)  [unwired: 1 in, 2 out]
      }
      event "STR_HostAddress": Key Down {
        n270 = event-data() -> ("VKey"=w582:T15)  [unwired: 1 in]
        n271 = Equal?(x=w582, y=eventvkey."Enter") -> (x = y?=w584:bool)
        n272 = Equal?(x=w582, y=eventvkey."Return") -> (x = y?=w585:bool)
        n273 = Or(x=w585, y=w584) -> (x .or. y?=w583:bool)
        n274 = case shown="True" w583 {
          tunnel: w581 -> [_ w591]
          tunnel: [w588 w590] -> w579
          tunnel: w580 -> [w588 w589]
          frame False {
          }
          frame True {
            n275 = Enqueue Element(queue=w591, element=Enum_MainQueueElements."Button_Connect_Pressed", error in (no error)=w589) -> (error out=w590:errorcluster)  [unwired: 1 in, 2 out]
          }
        }
      }
      event "Button_Disconnect": Value Change {
        n276 = event-data() -> ()  [unwired: 1 in, 3 out]
        n277 = Enqueue Element(queue=w595, element=Enum_MainQueueElements."Button_Disconnect_Pressed", error in (no error)=w594) -> (error out=w593:errorcluster)  [unwired: 1 in, 2 out]
      }
      event "LBox_ChList": Drag Starting? {
        n278 = event-data() -> ("CtlRef"=w603:refnum<vi>)  [unwired: 1 in]
        n279 = property on="Property Node" class="MCListbox (strict)"(reference=w603) -> ("Value"=w600:i32, "ItemNames"=w597:string[][])  [unwired: 1 in, 2 out]
        n280 = Index Array(array=w597, index (row)=w600, index (col)=0 ("disabled index (col)")) -> (element=w598:string)
        n281 = To Variant(anything=w598) -> (Variant=w606:variant)
        n282 = Bundle("DragChannel", "Variant"=w606) -> (w604:cluster{string, "Variant":variant})  [unwired: 1 in]
        n283 = Build Array(w604) -> (w601:cluster{string, "Variant":variant}[])
        n284 = event-data("Data"=w601, "Drag Mode"=enum32{"copy or move", "copy only", "move only"}."copy only") -> ()  [unwired: 1 in, 1 out]
      }
      event "STR_ChName1", "STR_ChName2", "STR_ChName3", "STR_ChName4", "STR_ChName5", "STR_ChName6", "STR_LoggingChName1", "STR_LoggingChName2", "STR_LoggingChName3", "STR_LoggingChName4", "STR_LoggingChName5", "STR_LoggingChName6": Drag Enter {
        n285 = event-data() -> ("Available Data Names"=w609:string[])  [unwired: 1 in, 1 out]
        n286 = Search 1D Array(1D array=w609, element="DragChannel") -> (index of element=w610:i32)  [unwired: 1 in]
        n287 = Greater Or Equal To 0?(x=w610) -> (x >= 0?=w607:bool)
        n288 = event-data("Accepted?"=w607) -> ()  [unwired: 1 in, 1 out]
      }
      event "STR_ChName1", "STR_ChName2", "STR_ChName3", "STR_ChName4", "STR_ChName5", "STR_ChName6", "STR_LoggingChName1", "STR_LoggingChName2", "STR_LoggingChName3", "STR_LoggingChName4", "STR_LoggingChName5", "STR_LoggingChName6": Drop {
        w621 = "DragChannel"
        n289 = event-data() -> ("CtlRef"=w616:refnum<vi>, "Available Data Names"=w620:string[])  [unwired: 1 in]
        n290 = Search 1D Array(1D array=w620, element=w621) -> (index of element=w622:i32)  [unwired: 1 in]
        n291 = case shown="Default" w622 {
          tunnel: w621 -> [_ w628]
          tunnel: [FALSE TRUE] -> w619
          tunnel: [" " w625] -> w617
          frame Default {
          }
          frame 0.. {
            n292 = Get Drag Drop Data(8:"", 9:w628) -> (3:w625:string)  [unwired: 1 in, 1 out]
          }
        }
        n293 = call "FGV_DrapAndDrop_Data.vi"("Modes"=TD_Case_SimpleFGVModes."Set", "error in (no error)"=w613, "Target String Element Ref"=w616, "Channel Name"=w617) -> ("error out"=w614:errorcluster)  [unwired: 5 in, 2 out]
        n294 = Enqueue Element(queue=w611, element=Enum_MainQueueElements."NewDragAndDrop", error in (no error)=w614) -> (error out=w612:errorcluster)  [unwired: 1 in, 2 out]
        n295 = event-data("Accepted?"=w619) -> ()  [unwired: 1 in, 1 out]
      }
      event Application Instance Close {
        n296 = event-data() -> ()  [unwired: 1 in, 4 out]
        n297 = Enqueue Element(queue=w631, element=Enum_MainQueueElements."CloseApp", error in (no error)=w629) -> ()  [unwired: 1 in, 3 out]
      }
    }
  }
  "Recorder" <- w4
  "RecoderLogging" <- w4
